vi "eyecat MAX v01.vi"() -> ()   [LabVIEW 2011]
doc: "This VI is an upgrade from the WIN 1_v4 that implements the ageing subrutine"
uses:
  Buttons/String output.ctl
  <vilib>/Utility/miscctls.llb/LVRowAndColumnTypeDef.ctl
  Buttons/Numeric control.ctl
  Buttons/String input.ctl
  Buttons/Numeric indicator.ctl
  Controls Win/Control 3.ctl
  <vilib>/Platform/TimedLoop/XDataNode/nitl_modes.ctl
  <vilib>/Platform/TimedLoop/XDataNode/timing_clust.ctl
  <vilib>/Platform/TimedLoop/XDataNode/wakeup.ctl
  <vilib>/Utility/file.llb/Write To Spreadsheet File (string).vi
  <vilib>/Utility/file.llb/Read From Spreadsheet File (string).vi
  <vilib>/Platform/TimedLoop/XDataNode/XDataNode.xnode
  <vilib>/regexp/Match Regular Expression.xnode
  <vilib>/Platform/TimedLoop/XDataNode/XDNodeRunTimeDep.lvlib
panel:
  out "Furnace temp 2":dbl
  out "output cluster":T2
  out "Full system?":bool
  out "Log interval (seconds)":T1
  in  "Flow rate Age":dbl
  in  "Inlet temp Age":dbl
  out "Stopped?":bool
  in  "Stop Cmd":T1
  out "Connected?":bool
  out "Error":dbl
  out "Iteration Duration":i64
  out "Finished Late? [i-1]":bool
  in  "stop TCP":bool
  in  "SO2 ppm":dbl
  out "Furnace temp 1":dbl
  out "stop 2":bool
  in  "Enum 1":i16=1
  in  "Acknowledge":bool
  out "Test number":u16
  out "Flag1":bool=TRUE
  out "EditPos Subc":T3
  out "Flag 2":bool=TRUE
  in  "Tab Control":T4(tab)
  out "Doors Unlocked":bool
  in  "Temperature Limit (°C)":T1=800.0 min=0.0 max=1200.0 step=1.0
  in  "Log Test Button":bool
  in  "File Name":T5
  in  "File Path":path=path "C:/DATA LOG"
  out "Fail":bool
  out "Pass":bool
  in  "Select Test Type":T6(radio)
  out "Standby":bool
  out "Doors Open":bool
  out "Extractor Fan On":bool
  out "Test In Progress":bool
  out "Cool Down":bool
  out "System Alarm":bool
  in  "Execute Leak Test Button":bool
  in  "Stop Test Button":bool
  in  "Start Test Button":bool
  in  "Advanced settings":bool
  in  "Inlet Temperature (°C)":T1=400.0 min=350.0 max=1000.0 step=1.0
  in  "Inlet LAMBDA Rich":T1=0.9 min=0.85 max=0.96 step=0.001
  in  "Inlet LAMBDA Lean":T1=1.2 min=1.02 max=3.0 step=0.001
  in  "Test Stop temperature (°C)":T1=300.0 min=100.0 max=1000.0 step=1.0
  in  "Test Start Temperature (°C)":T1=125.0 min=0.0 max=500.0 step=1.0
  in  "Furnace Ramp Rate (°C/min)":T1=15.0 min=1.0 max=50.0 step=0.1
  in  "NO:CO Ratio":T1=1.1 min=1.0 max=5.0 step=0.1
  in  "Inlet O2 (%)":T1=0.5 min=0.0 max=14.0 step=0.01
  in  "Inlet LAMBDA":T1=1.0 min=0.6 max=3.0 step=0.001
  out "Space Velocity (h-1)":T7
  out "Vol Flow @ STP (l/min)":T7
  in  "Test Flow Rate(g/s)":T1 min=0.0 max=100.0 step=0.01
  out "Sample Volume (litres)":T7
  in  "Number of Samples":T1=1.0 min=1.0 max=6.0 step=1.0
  in  "Sample Diameter (mm)":T1
  out "CO Theory (%)":T7 format="%#_3g"
  out "CO Theory (%)":T7 format="%#_3g"
  out "HC Theory (%)":T7
  in  "Sample Length (mm)":T1 min=0.0 step=0.5
  in  "NO ppm SW":dbl=500.0 caption="NO (ppm)" min=0.0 max=500.0 step=1.0
  in  "NO ppm Loff":T1 caption="NO ppm"
  in  "Delete sCycle":bool
  in  "Load sCycle":bool
  in  "Save sCycle":bool
  in  "Clear subcycle":bool
  in  "Clear Cycle Pattern":bool
  in  "Save Cycle":bool
  in  "Load Cycle":bool
  in  "Delete Cycle":bool
  out "Test Compiled":bool
  in  "Compile Test Button":bool
  in  "Sub-Cycle List":i32(listbox)=1
  in  "Cycle List":i32(listbox)=2
  out "Total Test Duration (hrs)":T8
  in  "Ageing Gas":enum32{"Radio Selection 1", "Radio Selection 2"}(radio)
  in  "Sub-Cycle Pattern":string[][](table) caption="Subcycle pattern"
  in  "Total Number of Cycles":T1=1.0 min=1.0 max=10000.0 step=1.0
  in  "Cycle Pattern":string[][](table)
  in  "Sub-Cycle Name":T5
  in  "Cycle Name":T5
  out "Heat Exchanger Temperatures (°C)":dynamicdata(graph)
  out "Flow Rate (g/s)":dynamicdata(graph)
  out "Sample Temperatures (°C)":dynamicdata(graph)
  out "System Temperatures (°C)":dynamicdata(graph)
  out "HC Concentration (ppm)":dynamicdata(graph)
  out "Lambda":dynamicdata(graph)
  out "M584L Upstream & Downstream":dynamicdata(graph)
  out "NO Concentration (ppm)":dynamicdata(graph)
  in  "Purge System":bool
  in  "Alarm ack":bool
  in  "Clear log":bool
  out "Table":string[][](table)
  out "Soft Alarm":bool
  out "Hard Alarm":bool
  # "Test Type"
  # "Test Commands"
  # "System Indicators"
  # "Leak Test"
  # "Catalyst Specification"
  # "Lightoff Settings"
  # "Furnace Lightoff Settings"
  # "Sweep Settings"
  # "CO/HC Lightoff Settings"
  # "0.96 < lambda < 0.85"
  # "1.02< lambda < 1.6"
  # "350 < Tinlet < 1000"
  # "NO Lightoff Settings"
  # "Flow Specification"
  # "Cycle Compiled"
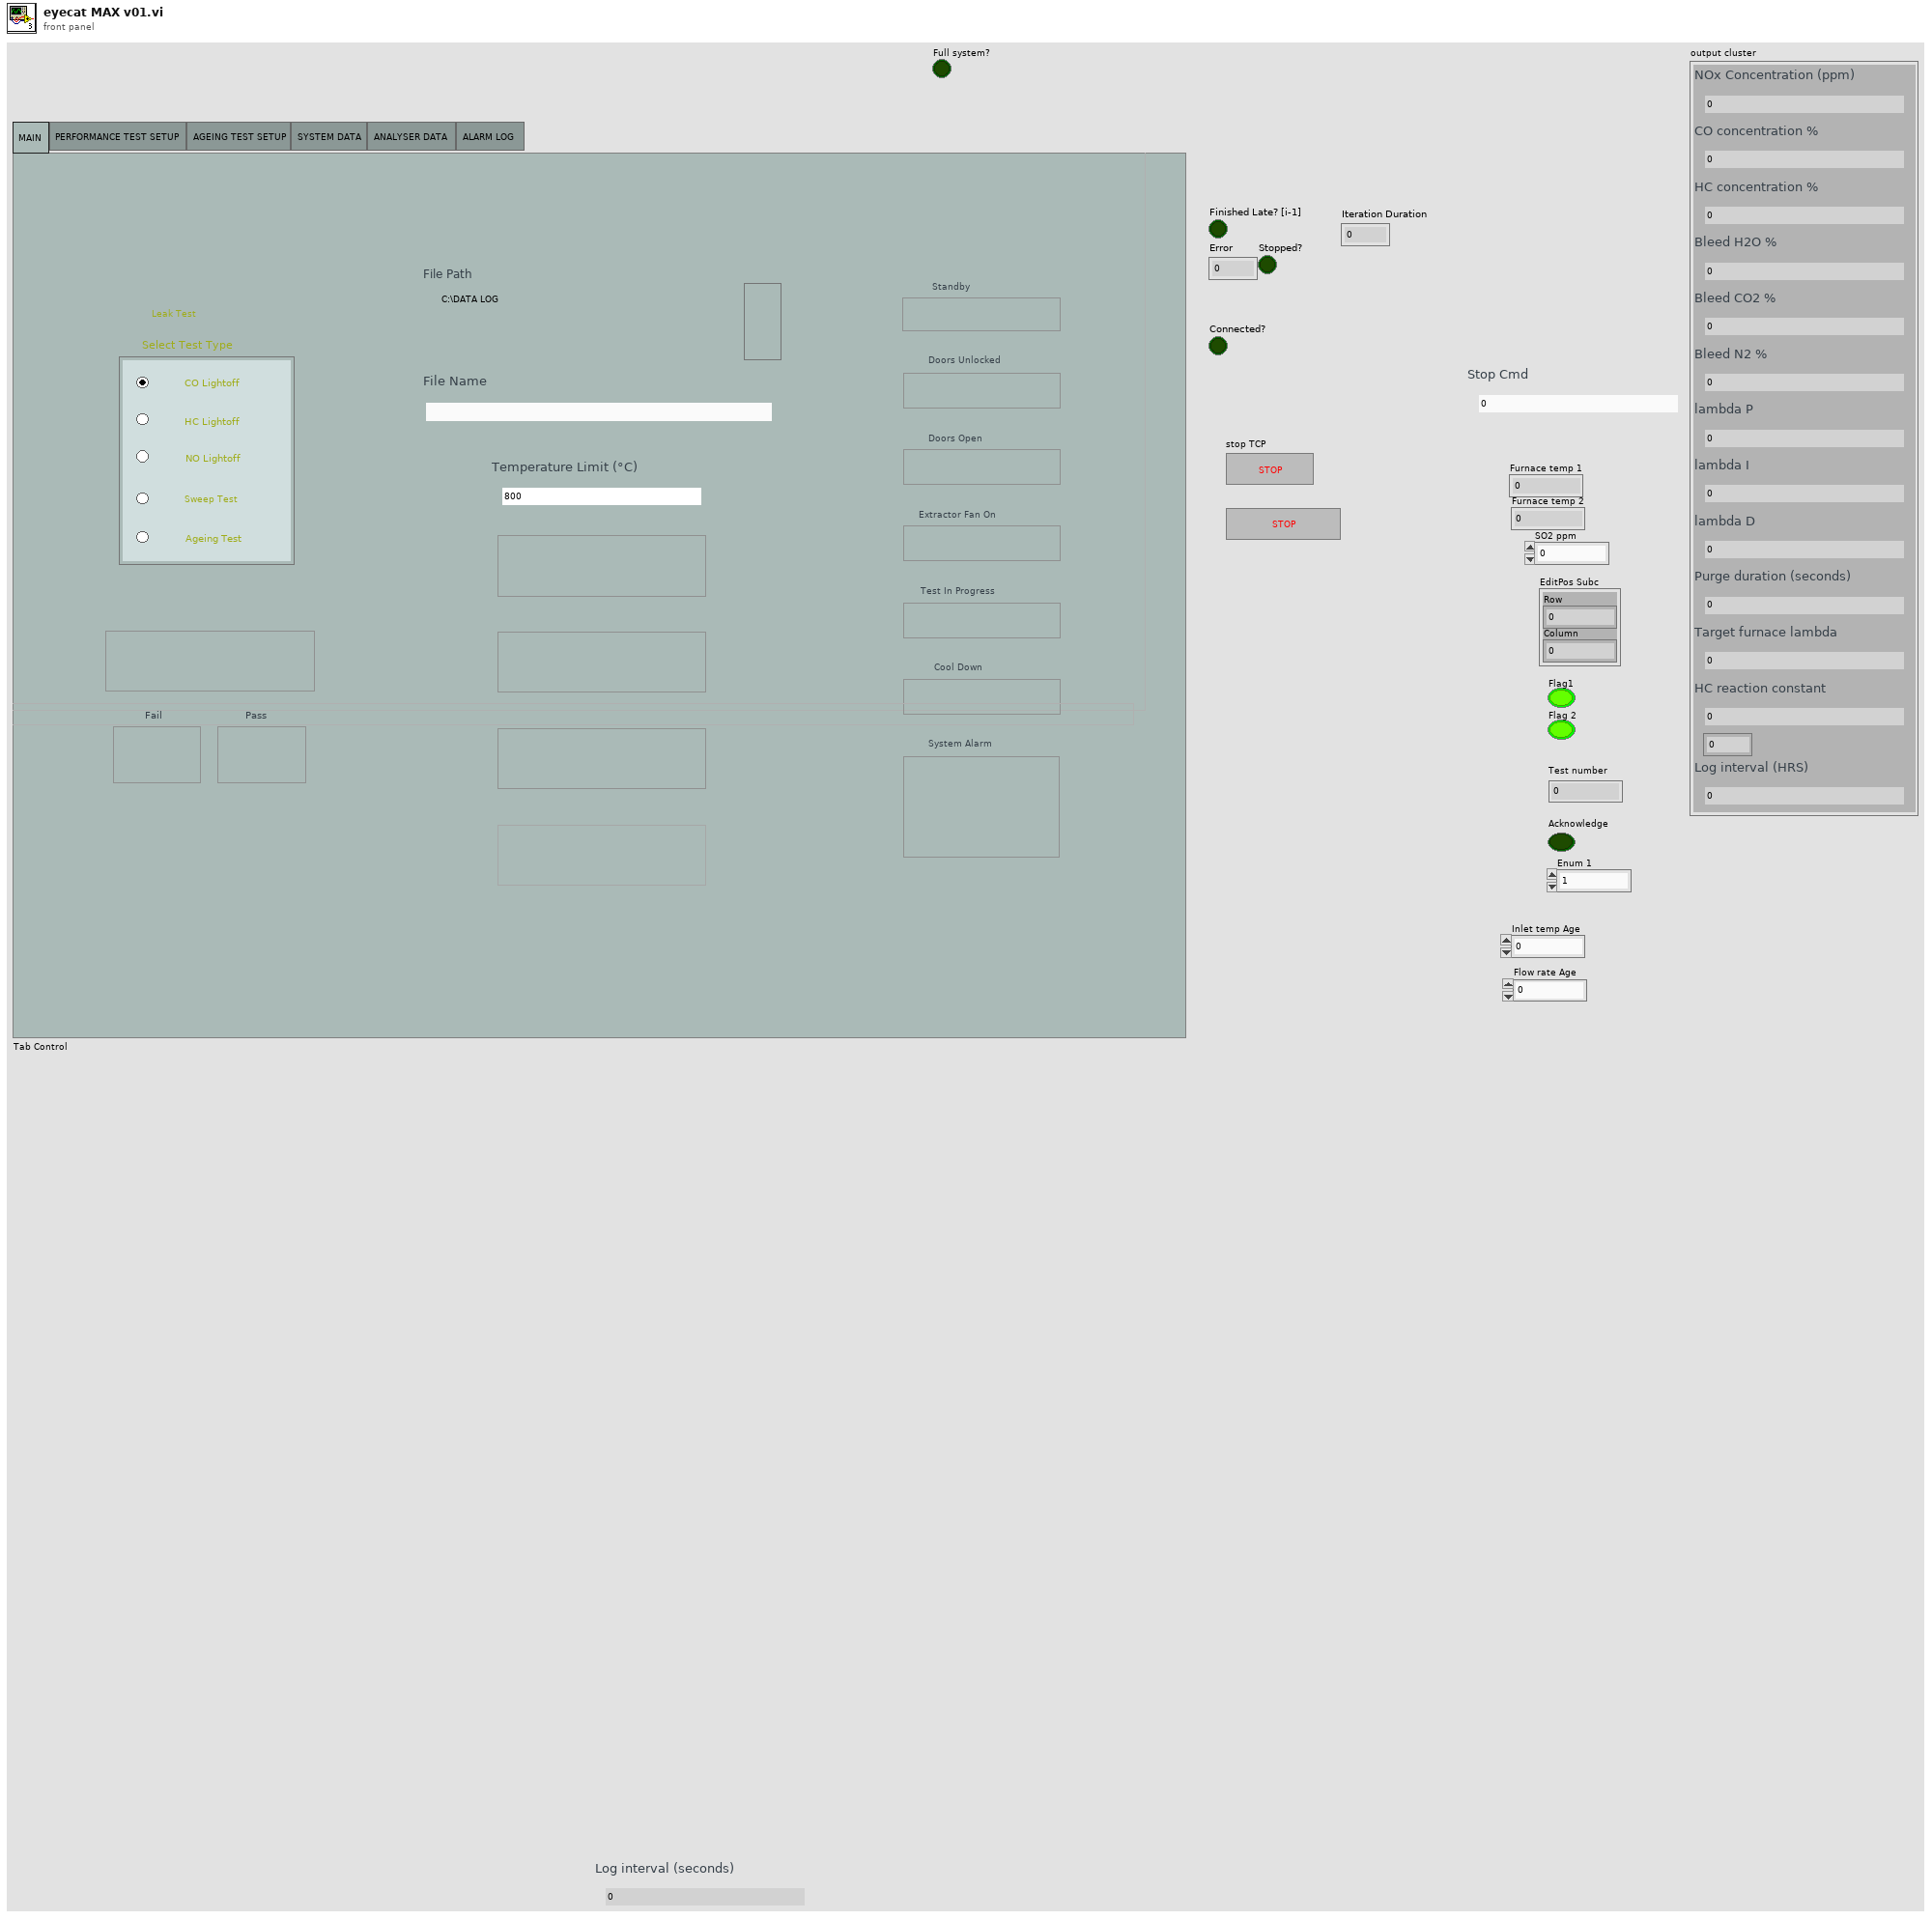
[diagram p1: front panel]
types:
  T1 = typedef "Numeric control.ctl" = dbl
  T2 = cluster{"NOx Concentration (ppm)":T1, "CO concentration %":T1, "HC concentration %":T1, "Bleed H2O %":T1, "Bleed CO2 %":T1, "Bleed N2 %":T1, "lambda P":T1, "lambda I":T1, "lambda D":T1, "Purge duration (seconds)":T1, "Target furnace lambda":T1, "HC reaction constant":T1, i16, "Log interval (HRS)":T1}
  T3 = typedef "LVRowAndColumnTypeDef.ctl" = cluster{"Row":i32, "Column":i32}
  T4 = enum32{"MAIN", "PERFORMANCE TEST SETUP", "AGEING TEST SETUP", "SYSTEM DATA", "ANALYSER DATA", "ALARM LOG"}
  T5 = typedef "String input.ctl" = string
  T6 = enum32{"CO Lightoff", "HC Lightoff", "NO Lightoff", "Sweep Test", "Ageing Test"}
  T7 = typedef "Numeric indicator.ctl" = dbl
  T8 = typedef "String output.ctl" = string
  T9 = typedef "XDNodeRunTimeDep.lvlib/nitl_modes.ctl" = enum32{"No Change", "Process missed periods, maintain original phase", "Discard missed periods, maintain original phase", "Process missed periods, ignore original phase", "Discard missed periods, ignore original phase"}
  T10 = typedef "Control 3.ctl" = enum16{"main", "start test", "save subc", "load subc", "delete subc", "clear table 1", "update list 1", "save cycle", "load cycle", "delete cycle", "clear table 2", "update list 2", "calc HC CO", "Total time calc", "update Cycle pattern ", "load cycle name", "convert to num", "load test array", "check scycle name", "check cycle name", "Multigas connect", "Multigas disconnect"}
  T11 = typedef "XDNodeRunTimeDep.lvlib/timing_clust.ctl" = cluster{"Expected End [f-1]":u64, "Actual End [f-1]":u64, "Finished Late? [f-1]":bool, "Expected End [i-1]":u64, "Actual End [i-1]":u64, "Finished Late? [i-1]":bool, "Expected Start [i]":u64, "Actual Start [i]":u64, "Expected Start [f]":u64, "Actual Start [f]":u64, "Source Name":string, "Structure Name":string, "Period":i64, "Deadline":i64, "Offset":i64, "Start":i64, "Priority":i32, "Timeout":i32, "Mode":T9, "Wakeup Reason":T12, "Error":errorcluster, "Source Type":string, "Secondary Source Type":string, "Global End Time":u64, "Global Start Time":u64, "Frame Duration":u64, "Iteration Duration":u64, "Assigned CPU":i32, "I/O Scan Engine Mode":u32}
  T12 = typedef "XDNodeRunTimeDep.lvlib/wakeup.ctl" = enum32{"Normal", "Aborted", "Asynchronous wakeup", "Timing source error", "Timed loop error", "Timeout"}
  T13 = enum8{"Enabled", "Disabled", "Disabled and Grayed Out"}
  T14 = cluster{"NOx Concentration (ppm)":T1, "CO concentration %":T1, "HC concentration %":T1, "Bleed H2O %":T1, "Bleed CO2 %":T1, "Bleed N2 %":T1, "lambda P":T1, "lambda I":T1, "lambda D":T1, "Purge duration (seconds)":T1, "Target furnace lambda":T1, "HC reaction constant":T1, "Full System?":i16, "Log interval (HRS)":T1}
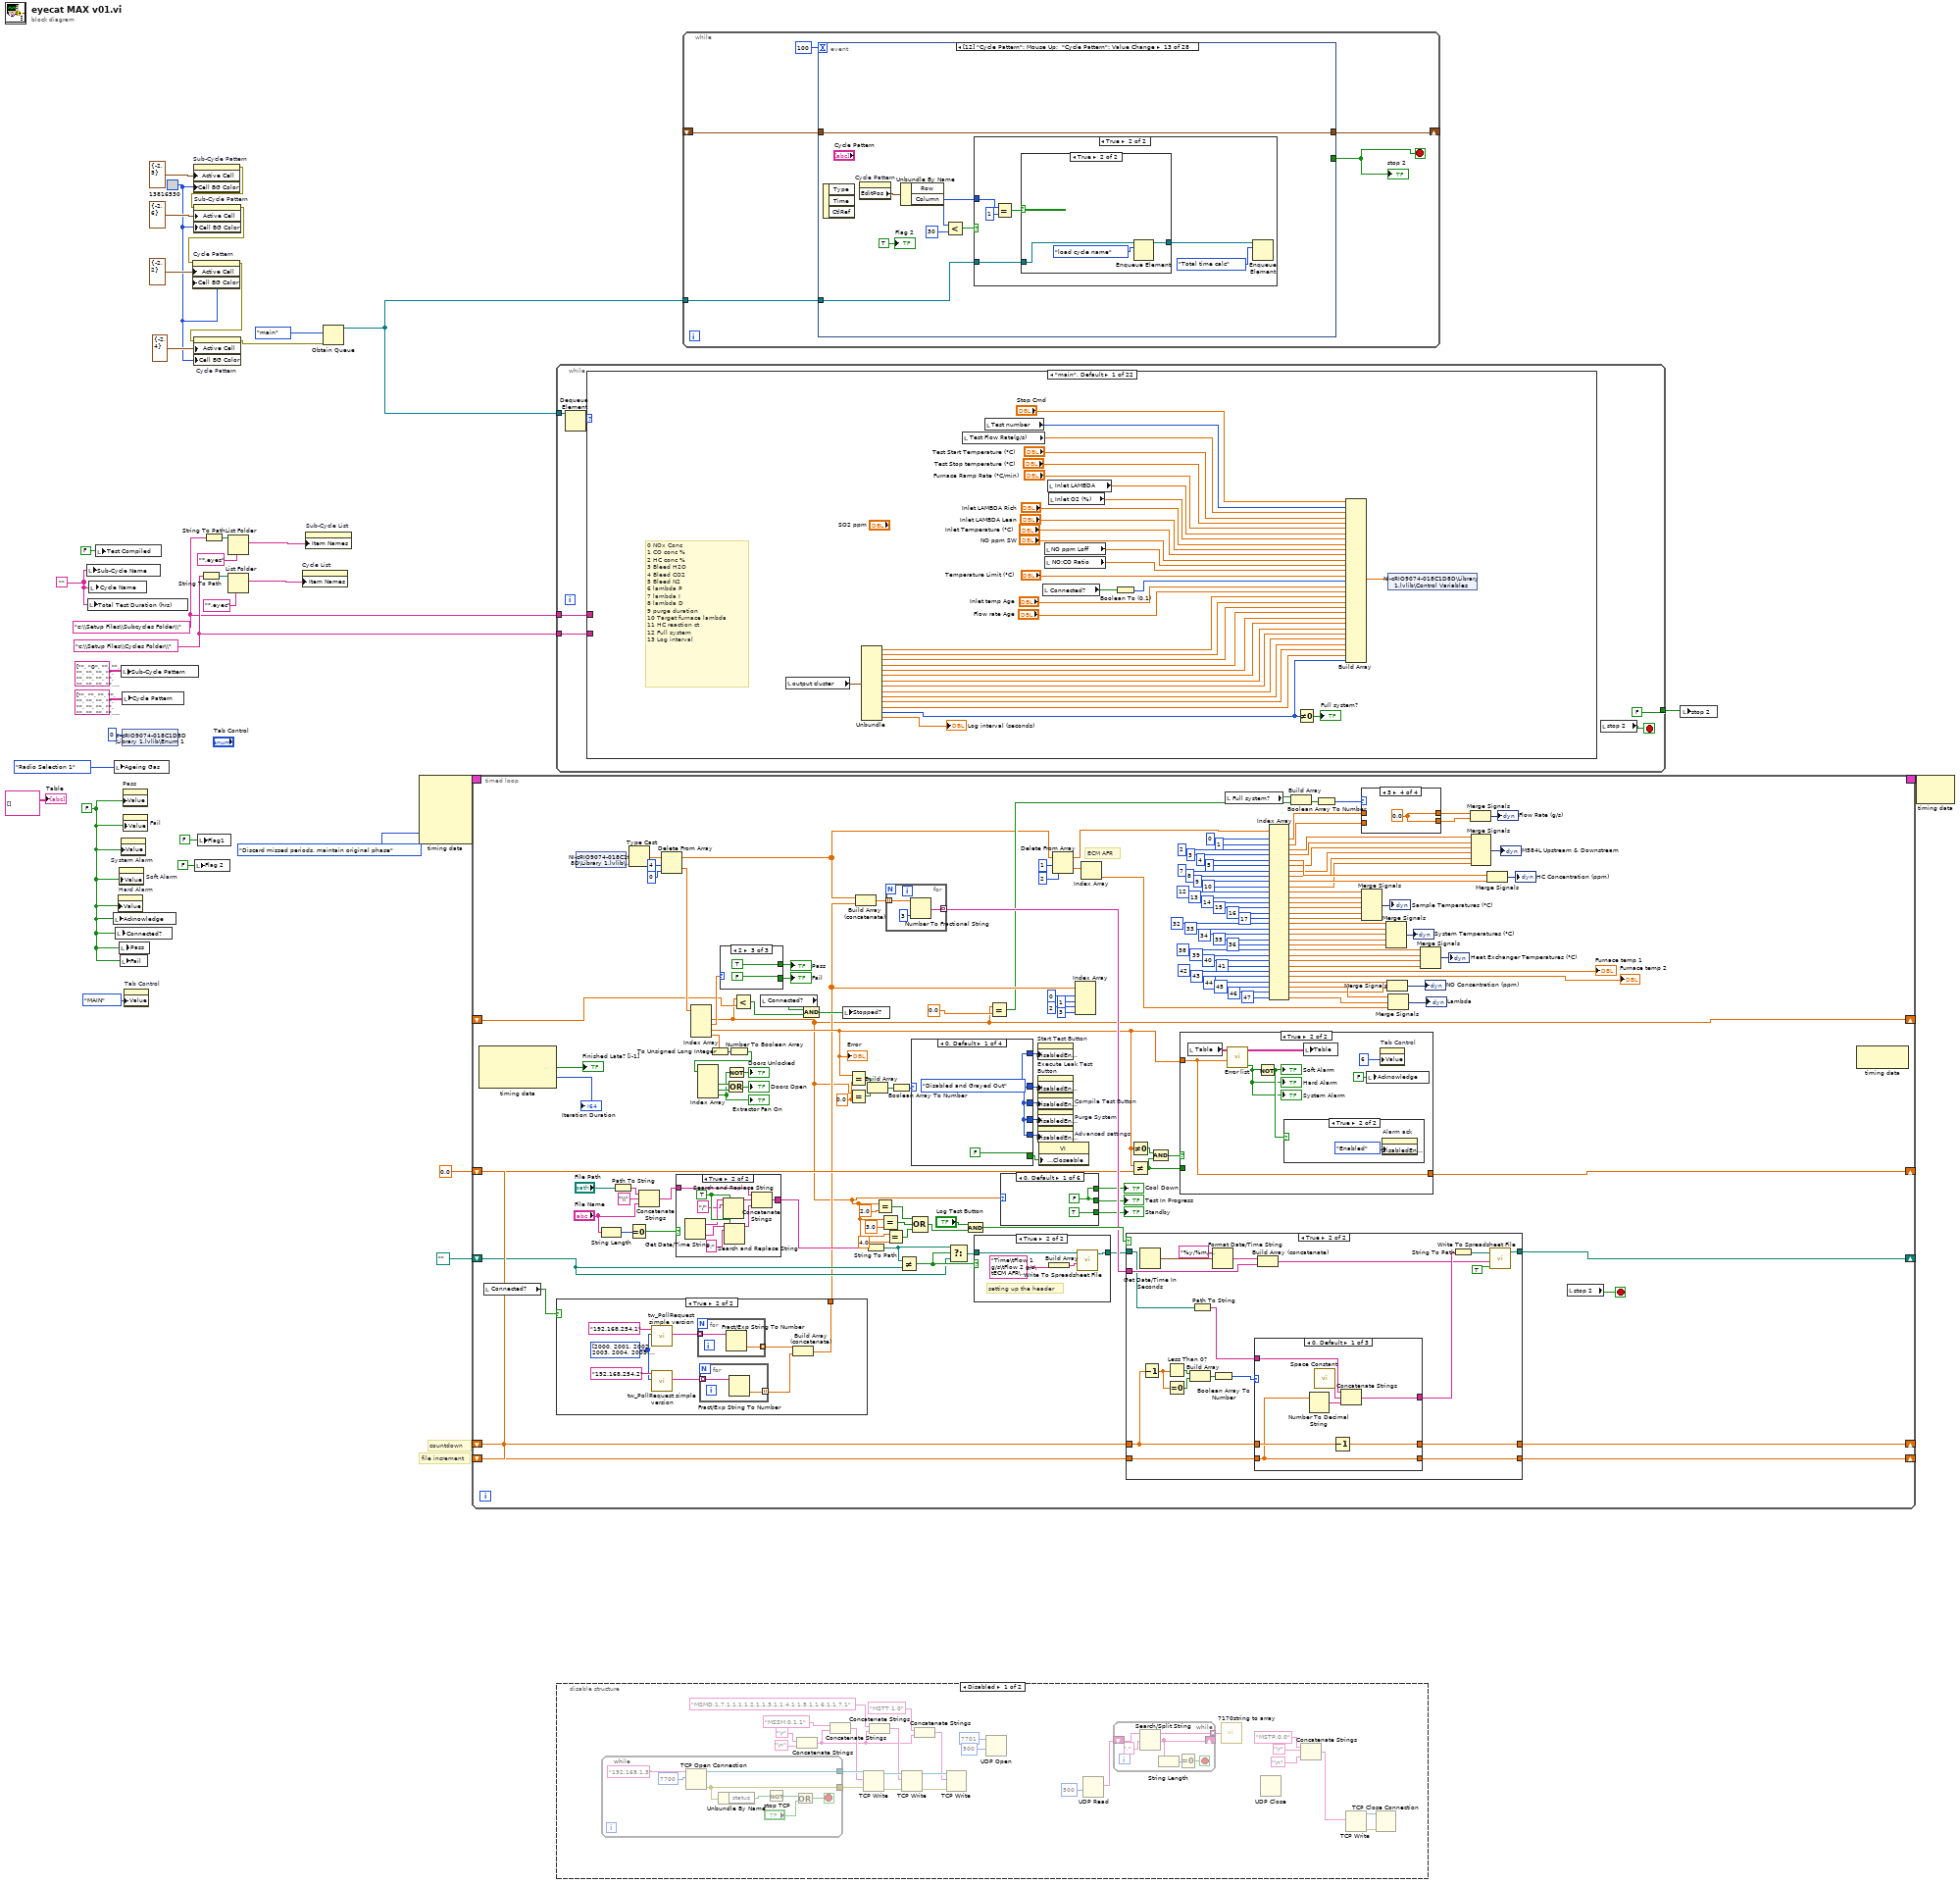
[diagram p0: block diagram]
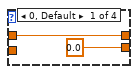
[diagram p3: hidden frame]
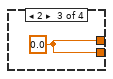
[diagram p5: hidden frame]
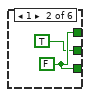
[diagram p7: hidden frame]
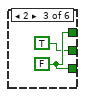
[diagram p8: hidden frame]
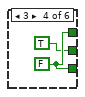
[diagram p9: hidden frame]
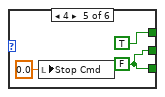
[diagram p10: hidden frame]
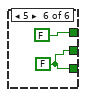
[diagram p11: hidden frame]
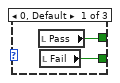
[diagram p12: hidden frame]
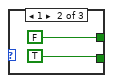
[diagram p13: hidden frame]
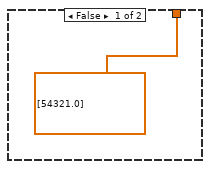
[diagram p14: hidden frame]
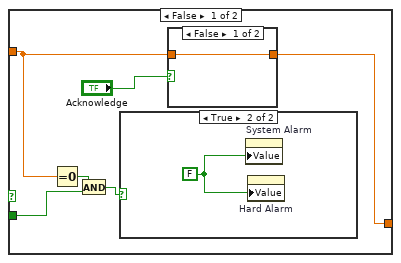
[diagram p15: hidden frame]
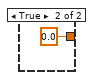
[diagram p16: hidden frame]
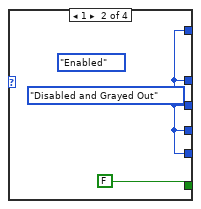
[diagram p19: hidden frame]
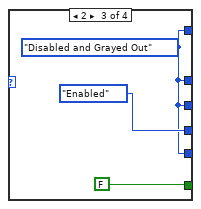
[diagram p20: hidden frame]
diagram:
  w2 = FALSE
  w1 = 0.0 ("y")
  w18 = ""
  w21 = "c:\\Setup Files\\Cycles Folder\\"
  w27 = u32 13816530
  w19 = "c:\\Setup Files\\Subcycles Folder\\"
  # "file increment"
  # "countdown"
  n1 = local write "Sub-Cycle Name"(w18) -> ()
  n2 = local write "Total Test Duration (hrs)"(w18) -> ()
  n3 = local write "Cycle Name"(w18) -> ()
  n4 = local write "Test Compiled"(FALSE ("Cycle Compiled")) -> ()
  n5 = local write "Acknowledge"(w2) -> ()
  n6 = local write "Ageing Gas"(enum32{"Radio Selection 1", "Radio Selection 2"}."Radio Selection 1" ("Ageing Gas")) -> ()
  n7 = local write "Connected?"(w2) -> ()
  n8 = property on="Hard Alarm" class="Bool (strict)"("Value"=w2) -> ()  [unwired: 2 in, 2 out]
  n9 = property on="Soft Alarm" class="Bool (strict)"("Value"=w2) -> ()  [unwired: 2 in, 2 out]
  n10 = local write "Pass"(w2) -> ()
  n11 = local write "Fail"(w2) -> ()
  n12 = local write "Sub-Cycle Pattern"(string[][] [["", "0", "", "", "", "", "", "", "", "", "", "", ""], ["", "", "", "", "", "", "", "", "", "", "", "", ""], ["", "", "", "", "", "", "", "", "", "", "", "", ""], ["", "", "", "", "", "", "", "", "", "", "", "", ""], ["", "", "", "", "", "", "", "", "", "", "", "", ""], ["", "", "", "", "", "", "", "", "", "", "", "", ""], ["", "", "", "", "", "", "", "", "", "", "", "", ""], ["", "", "", "", "", "", "", "", "", "", "", "", ""], ["", "", "", "", "", "", "", "", "", "", "", "", ""], ["", "", "", "", "", "", "", "", "", "", "", "", ""], ["", "", "", "", "", "", "", "", "", "", "", "", ""], ["", "", "", "", "", "", "", "", "", "", "", "", ""], ["", "", "", "", "", "", "", "", "", "", "", "", ""], ["", "", "", "", "", "", "", "", "", "", "", "", ""], ["", "", "", "", "", "", "", "", "", "", "", "", ""], ["", "", "", "", "", "", "", "", "", "", "", "", ""], ["", "", "", "", "", "", "", "", "", "", "", "", ""], ["", "", "", "", "", "", "", "", "", "", "", "", ""], ["", "", "", "", "", "", "", "", "", "", "", "", ""], ["", "", "", "", "", "", "", "", "", "", "", "", ""], ["", "", "", "", "", "", "", "", "", "", "", "", ""], ["", "", "", "", "", "", "", "", "", "", "", "", ""], ["", "", "", "", "", "", "", "", "", "", "", "", ""], ["", "", "", "", "", "", "", "", "", "", "", "", ""], ["", "", "", "", "", "", "", "", "", "", "", "", ""], ["", "", "", "", "", "", "", "", "", "", "", "", ""], ["", "", "", "", "", "", "", "", "", "", "", "", ""], ["", "", "", "", "", "", "", "", "", "", "", "", ""], ["", "", "", "", "", "", "", "", "", "", "", "", ""], ["", "", "", "", "", "", "", "", "", "", "", "", ""], ["", "", "", "", "", "", "", "", "", "", "", "", ""]]) -> ()
  n13 = property on="System Alarm" class="Bool (strict)"("Value"=w2) -> ()  [unwired: 2 in, 2 out]
  n14 = local write "Cycle Pattern"(string[][] [["", "", "", "", ""], ["", "", "", "", ""], ["", "", "", "", ""], ["", "", "", "", ""], ["", "", "", "", ""], ["", "", "", "", ""], ["", "", "", "", ""], ["", "", "", "", ""], ["", "", "", "", ""], ["", "", "", "", ""], ["", "", "", "", ""], ["", "", "", "", ""], ["", "", "", "", ""], ["", "", "", "", ""], ["", "", "", "", ""], ["", "", "", "", ""], ["", "", "", "", ""], ["", "", "", "", ""], ["", "", "", "", ""], ["", "", "", "", ""], ["", "", "", "", ""], ["", "", "", "", ""], ["", "", "", "", ""], ["", "", "", "", ""], ["", "", "", "", ""], ["", "", "", "", ""], ["", "", "", "", ""], ["", "", "", "", ""], ["", "", "", "", ""], ["", "", "", "", ""], ["", "", "", "", ""]]) -> ()
  n15 = shared-variable "NI-cRIO9074-018C1D8D\\Library 1.lvlib\\Enum 1"(u16 0 ("Enum 1")) -> ()  [unwired: 1 in, 1 out]
  n16 = property on="Pass" class="Bool (strict)"("Value"=w2) -> ()  [unwired: 2 in, 2 out]
  n17 = property on="Fail" class="Bool (strict)"("Value"=w2) -> ()  [unwired: 2 in, 2 out]
  n18 = property on="Tab Control" class="TabCtl (strict)"("Value"=T4."MAIN" ("Tab Control")) -> ()  [unwired: 2 in, 2 out]
  n19 = property on="Sub-Cycle Pattern" class="Tbl (strict)"("Active Cell"=T3 {"Row"=-2, "Column"=5} ("Active Cell:Active Cell"), "Cell BG Color"=w27) -> (error out=w32:errorcluster)  [unwired: 2 in, 1 out]
  n20 = property on="Sub-Cycle Pattern" class="Tbl (strict)"(error in=w32, "Active Cell"=T3 {"Row"=-2, "Column"=6} ("Active Cell:Active Cell"), "Cell BG Color"=w27) -> (error out=w31:errorcluster)  [unwired: 1 in, 1 out]
  n21 = property on="Cycle Pattern" class="Tbl (strict)"(error in=w31, "Active Cell"=T3 {"Row"=-2, "Column"=2} ("Active Cell:Active Cell"), "Cell BG Color"=w27) -> (error out=w29:errorcluster)  [unwired: 1 in, 1 out]
  n22 = property on="Cycle Pattern" class="Tbl (strict)"(error in=w29, "Active Cell"=T3 {"Row"=-2, "Column"=4} ("Active Cell:Active Cell"), "Cell BG Color"=w27) -> (error out=w26:errorcluster)  [unwired: 1 in, 1 out]
  n23 = local write "Flag 2"(FALSE) -> ()
  n24 = local write "Flag1"(FALSE) -> ()
  n25 = String To Path(string=w21) -> (path=w22:path)
  n26 = String To Path(string=w19) -> (path=w24:path)
  n27 = List Folder(path=w22, pattern="*.eyec") -> (filenames=w23:string[])  [unwired: 2 in, 3 out]
  n28 = List Folder(path=w24, pattern="*.eyes") -> (filenames=w25:string[])  [unwired: 2 in, 3 out]
  n29 = property on="Cycle List" class="LstBox (strict)"("Item Names"=w23) -> ()  [unwired: 2 in, 2 out]
  n30 = property on="Sub-Cycle List" class="LstBox (strict)"("Item Names"=w25) -> ()  [unwired: 2 in, 2 out]
  n31 = Obtain Queue(element data type=Control_3."main" ("Enum"), error in (no error)=w26) -> (queue out=w35:refnum<queue>)  [unwired: 3 in, 2 out]
  n32 = node-c288(nitl_modes."Discard missed periods, maintain original phase" ("Mode")) -> (w7:T11)  [unwired: 4 in]
  n33 = timed-loop {
    timing: w7 -> [_]
    timing-out: [_] -> w6
    shift-right: [w168] -> _
    shift-left: path "" -> [w170]
    shift-right: [w119] -> _
    shift-left: w1 -> [w169]
    shift-right: [w38] -> _
    shift-left: _ -> [w133]
    shift-right: [w108] -> _
    shift-left: w1 -> [w112]
    shift-right: [w109] -> _
    shift-left: w1 -> [w111]
    stop <- w167 stop-if-true
    w150 = 0.0 ("y")
    # "ECM AFR"
    n34 = node-c288() -> (→"Finished Late? [i-1]":bool, →"Iteration Duration":i64)  [unwired: 1 in, 1 out]
    n35 = local read "Connected?"() -> (w156:bool)
    n36 = case shown="True" w156 {
      tunnel: [dbl[] [54321.0] ("Output") w235] -> w107
      frame False {
      }
      frame True {
        w238 = i32[] [2000, 2001, 2002, 2003, 2004, 2005, 2006, 2007, 2008, 2009, 2010, 2011, 2012, 2013, 2014] ("EVID list")
        n37 = call <userlib>:"tw_PollRequest simple version.vi"("EVID list"=w238, "IP_ADD [127.0.0.1]"="192.168.254.1") -> ("values out"=w241:string[])  [unwired: 7 in, 2 out]
        n38 = call <userlib>:"tw_PollRequest simple version.vi"("EVID list"=w238, "IP_ADD [127.0.0.1]"="192.168.254.2") -> ("values out"=w240:string[])  [unwired: 7 in, 2 out]
        n39 = for {
          tunnel: [w246] -> w236 mode=indexing
          tunnel: w241 -> [w245] mode=indexing
          n40 = Fract/Exp String To Number(string=w245) -> (number=w246:dbl)  [unwired: 3 in, 1 out]
        }
        n41 = for {
          tunnel: [w244] -> w237 mode=indexing
          tunnel: w240 -> [w243] mode=indexing
          n42 = Fract/Exp String To Number(string=w243) -> (number=w244:dbl)  [unwired: 3 in, 1 out]
        }
        n43 = Build Array (concatenate)(w236, w237) -> (w235:dbl[])
      }
    }
    n44 = shared-variable "NI-cRIO9074-018C1D8D\\Library 1.lvlib\\DATA"() -> (w166:dbl[])  [unwired: 1 in, 1 out]
    n45 = String Length(string="File Name") -> (length=w124:i32)
    n46 = Path To String(path="File Path") -> (string=w126:string)
    n47 = Equal To 0?(x=w124) -> (x = 0?=w122:bool)
    n48 = Type Cast(type=w166, x=w166) -> (*(type *) &x=w179:dbl[])
    n49 = Concatenate Strings(w126, "\\" ("string"), "File Name") -> (w121:string)
    n50 = Delete From Array(array=w179, length=4, index=0) -> (deleted portion=w176:dbl[], array with subset deleted=w48:dbl[])
    n51 = case shown="True" w122 {
      tunnel: [w205 w213] -> w110
      tunnel: w121 -> [w205 w214]
      frame False {
      }
      frame True {
        w211 = TRUE ("replace all? (F)")
        n52 = Get Date/Time String() -> (date string=w209:string, time string=w210:string)  [unwired: 3 in]
        n53 = Search and Replace String(replace all?=w211, input string=w209, search string="/") -> (result string=w212:string)  [unwired: 5 in, 3 out]
        n54 = Search and Replace String(replace all?=w211, input string=w210, search string=":") -> (result string=w206:string)  [unwired: 5 in, 3 out]
        n55 = Concatenate Strings(w214, w212, w206) -> (w213:string)
      }
    }
    n56 = Index Array(array=w176) -> (element #1=w38:dbl, element #2=w139:dbl, element #3=w140:dbl, element #4=w132:dbl)  [unwired: 4 in]
    "Error" <- w140
    n57 = To Unsigned Long Integer(number=w132) -> (unsigned 32bit integer=w131:u32)
    n58 = case shown="2" w139 {
      tunnel: [w228 TRUE FALSE] -> w138
      tunnel: [w229 FALSE TRUE] -> w137
      frame 0, Default {
        n59 = local read "Pass"() -> (w229:bool)
        n60 = local read "Fail"() -> (w228:bool)
      }
      frame 1 {
      }
      frame 2 {
      }
    }
    "Pass" <- w137
    "Fail" <- w138
    n61 = Number To Boolean Array(number=w131) -> (Boolean array=w155:bool[])
    n62 = Index Array(array=w155) -> (element #2=w153:bool, element #3=w152:bool, element #4=w128:bool)  [unwired: 4 in, 1 out]
    "Extractor Fan On" <- w128
    n63 = Or(x=w153, y=w152) -> (x .or. y?=→"Doors Open":bool)
    n64 = Not(x=w128) -> (.not. x?=→"Doors Unlocked":bool)
    n65 = Less?(x=w38, y=w133) -> (x < y?=w130:bool)
    n66 = local read "Connected?"() -> (w129:bool)
    n67 = And(x=w129, y=w130) -> (x .and. y?=w118:bool)
    n68 = local write "Stopped?"(w118) -> ()
    n69 = Equal?(x=w140, y=w150) -> (x = y?=w148:bool)
    n70 = Equal?(x=w38, y=w150) -> (x = y?=w147:bool)
    n71 = Build Array (concatenate)(w48, w107) -> (w172:dbl[])
    n72 = String To Path(string=w110) -> (path=w120:path)
    n73 = Build Array(w148, w147) -> (w146:bool[])
    n74 = Equal?(x=w38, y=2.0) -> (x = y?=w50:bool)
    n75 = Equal?(x=w38, y=3.0) -> (x = y?=w41:bool)
    n76 = Equal?(x=w38, y=4.0) -> (x = y?=w39:bool)
    n77 = for {
      tunnel: w172 -> [w279] mode=indexing
      tunnel: [w278] -> w183 mode=indexing
      n78 = Number To Fractional String(number=w279, precision (6)=i16 3) -> (F-format string=w278:string)  [unwired: 2 in]
    }
    n79 = Boolean Array To Number(Boolean array=w146) -> (number=w145:u32)
    n80 = Not Equal?(x=w120, y=w170) -> (x != y?=w181:bool)
    n81 = case shown="0, Default" w145 {
      tunnel: [w265 w267 w269 w272] -> w149
      tunnel: [w265 w267 w269 w272] -> w144
      tunnel: [w265 w267 w269 w272] -> w143
      tunnel: [w265 w267 T13."Enabled" ("Disabled") w272] -> w142
      tunnel: [w265 w267 w269 w272] -> w141
      tunnel: [FALSE FALSE FALSE TRUE] -> w117
      frame 0, Default {
        w265 = T13."Disabled and Grayed Out" ("Disabled")
      }
      frame 1 {
        (unwired) T13."Enabled" ("Disabled")
        w267 = T13."Disabled and Grayed Out" ("Disabled")
      }
      frame 2 {
        w269 = T13."Disabled and Grayed Out" ("Disabled")
      }
      frame 3 {
        w272 = T13."Enabled" ("Disabled")
        (unwired) T13."Disabled and Grayed Out" ("Disabled")
      }
    }
    n82 = Compound Arithmetic op=OR(w50, w41, w39) -> (w49:bool)
    n83 = Select(t=w120, s=w181, f=w170) -> (s? t:f=w182:path)
    n84 = And(x="Log Test Button", y=w49) -> (x .and. y?=w198:bool)
    n85 = case shown="True" w181 {
      tunnel: w182 -> [w273 w277]
      tunnel: [w273 w276] -> w180
      frame False {
      }
      frame True {
        # "setting up the header"
        n86 = Build Array("Time\tFlow 1 g/s\tFlow 2 g/s\tECM AFR\tCO2 U %\tCO U %\tHC U ppm\tO2 U %\tNO U ppm\tCO2 D %\tCO D %\tHC D ppm\tO2 D %\tNO D ppm\tTC1X\tTC2A\tTCY\tTC4B\tTC5\tTC6\tTC7\tTC8\tTC9\tTC10\tTC11\tTC12\tTC13\tTC14\tTC15\tTC16\tTC17\tTC18\tTC19\tTC20\tTC Vent 1\tTC Vent 2\tTC Fan B1\tTC Fan B2\tTC Cab\tTC Ex A\tTC Ex B\tTC Ex C\tTC Ex D\tTC Furn 1\tTC Furn 2\tNOX 1 ppm\tNLambda 1\tNOX 2 ppm\tNLambda 2\tEGO 1\tEGO 2\tEGO 3\tEGO 4\tCO2 U %\tCO U %\tHC U ppm\tO2 U %\tNO U ppm\tCO2 D %\tCO D %\tHC D ppm\tO2 D %\tNO D ppm\r\n" ("Heading string 2")) -> (w275:string[])
        n87 = call-poly <vilib>:"Write To Spreadsheet File.vi"("1D data"=w275, "file path (dialog if empty)"=w277) -> ("new file path (Not A Path if cancelled)"=w276:path)  [unwired: 6 in]
      }
    }
    n88 = Equal?(x=w38, y=0.0) -> (x = y?=w104:bool)
    n89 = case shown="0, Default" w38 {
      tunnel: [w215 w218 w220 w222 TRUE FALSE] -> w136
      tunnel: [w215 TRUE TRUE TRUE w224 w226] -> w135
      tunnel: [TRUE w218 w220 w222 w224 w226] -> w134
      frame 0, Default {
        w215 = FALSE
      }
      frame 1 {
        w218 = FALSE
      }
      frame 2 {
        w220 = FALSE
      }
      frame 3 {
        w222 = FALSE
      }
      frame 4 {
        w224 = FALSE
        n90 = local write "Stop Cmd"(T1 0.0 ("Stop Cmd")) -> ()
      }
      frame 5 {
        w226 = FALSE
      }
    }
    "Cool Down" <- w136
    "Test In Progress" <- w135
    "Standby" <- w134
    n91 = property on="Start Test Button" class="Bool"("DisabledEnum"=w149) -> ()  [unwired: 2 in, 2 out]
    n92 = property on="Execute Leak Test Button" class="Bool"("DisabledEnum"=w144) -> ()  [unwired: 2 in, 2 out]
    n93 = property on="Compile Test Button" class="Bool"("DisabledEnum"=w143) -> ()  [unwired: 2 in, 2 out]
    n94 = property on="Purge System" class="Bool"("DisabledEnum"=w142) -> ()  [unwired: 2 in, 2 out]
    n95 = property on="Advanced settings" class="Bool"("DisabledEnum"=w141) -> ()  [unwired: 2 in, 2 out]
    n96 = property class="VI"("Front Panel.Closeable"=w117) -> ()  [unwired: 2 in, 2 out]
    n97 = Delete From Array(array=w48, length=1, index=2) -> (deleted portion=w45:dbl[], array with subset deleted=w43:dbl[])
    n98 = Index Array(array=w107, index #1=0 ("index"), index #2=1 ("index"), index #3=2 ("index"), index #4=3 ("index")) -> ()  [unwired: 4 out]
    n99 = Index Array(array=w45) -> (element=w44:dbl)  [unwired: 1 in]
    n100 = case shown="True" w198 {
      tunnel: w180 -> [w283 w291]
      tunnel: [w283 w303] -> w168
      tunnel: w183 -> [_ w299]
      tunnel: w112 -> [_ w292]
      tunnel: w111 -> [w282 w287]
      tunnel: [w282 w289] -> w109
      tunnel: [w281 w288] -> w108
      frame False {
        n101 = local read "Log interval (seconds)"() -> (w281:T1)
      }
      frame True {
        n102 = Get Date/Time In Seconds() -> (seconds since 1Jan1904=w300:timestamp)
        n103 = Decrement(x=w292) -> (x-1=w293:T1)
        n104 = Less Than 0?(x=w293) -> (x < 0?=w294:bool)
        n105 = Equal To 0?(x=w293) -> (x = 0?=w295:bool)
        n106 = Build Array(w294, w295) -> (w296:bool[])
        n107 = Path To String(path=w291) -> (string=w286:string)
        n108 = Format Date/Time String(time format string (%c)="%y/%m/%d %H:%M:%S", seconds (now)=w300) -> (date/time string=w301:string)  [unwired: 1 in]
        n109 = Boolean Array To Number(Boolean array=w296) -> (number=w297:u32)
        n110 = case shown="0, Default" w297 {
          tunnel: w292 -> [w310 w311 _]
          tunnel: [w309 w311 w314] -> w288
          tunnel: w286 -> [w308 w313 w317]
          tunnel: [w305 w313 w315] -> w290
          tunnel: [w304 w312 w316] -> w289
          tunnel: w287 -> [w304 w312 w320]
          frame 0, Default {
            n111 = Number To Decimal String(number=w304) -> (decimal integer string=w306:string)  [unwired: 1 in]
            n112 = call <vilib>:"Space Constant.vi"() -> ("String"=w307:string)
            n113 = Decrement(x=w310) -> (x-1=w309:T1)
            n114 = Concatenate Strings(w308, w307, w306) -> (w305:string)
          }
          frame 1 {
          }
          frame 2 {
            n115 = local read "Log interval (seconds)"() -> (w314:T1)
            n116 = Increment(x=w320) -> (x+1=w316:dbl)
            n117 = Number To Decimal String(number=w316) -> (decimal integer string=w318:string)  [unwired: 1 in]
            n118 = call <vilib>:"Space Constant.vi"() -> ("String"=w319:string)
            n119 = Concatenate Strings(w317, w319, w318) -> (w315:string)
          }
        }
        n120 = Build Array (concatenate)(w301, w299) -> (w285:string[])
        n121 = String To Path(string=w290) -> (path=w284:path)
        n122 = call-poly <vilib>:"Write To Spreadsheet File.vi"("append to file? (new file:F)"=TRUE, "1D data"=w285, "file path (dialog if empty)"=w284) -> ("new file path (Not A Path if cancelled)"=w303:path)  [unwired: 5 in]
      }
    }
    n123 = Not Equal To 0?(x=w140) -> (x != 0?=w174:bool)
    n124 = Not Equal?(x=w140, y=w169) -> (x != y?=w173:bool)
    n125 = And(x=w174, y=w173) -> (x .and. y?=w175:bool)
    n126 = case shown="True" w175 {
      tunnel: w140 -> [w248 w259]
      tunnel: w173 -> [w251 _]
      tunnel: [w247 w259] -> w119
      frame False {
        n127 = Equal To 0?(x=w248) -> (x = 0?=w252:bool)
        n128 = And(x=w252, y=w251) -> (x .and. y?=w250:bool)
        n129 = case shown="True" w250 {
          frame False {
          }
          frame True {
            w255 = FALSE ("Ack hard alarm!")
            n130 = property on="System Alarm" class="Bool (strict)"("Value"=w255) -> ()  [unwired: 2 in, 2 out]
            n131 = property on="Hard Alarm" class="Bool (strict)"("Value"=w255) -> ()  [unwired: 2 in, 2 out]
          }
        }
        n132 = case shown="False" "Acknowledge" {
          tunnel: [w253 0.0 ("Numeric")] -> w247
          tunnel: w248 -> [w253 _]
          frame False {
          }
          frame True {
          }
        }
      }
      frame True {
        n133 = local read "Table"() -> (w262:string[][])
        n134 = call "Error list.vi"("Error code"=w259, "Error array in"=w262) -> ("Hard alarm?"=w256:bool, "Error array out"=w261:string[][])  [unwired: 8 in]
        "Hard Alarm" <- w256
        "System Alarm" <- w256
        n135 = Not(x=w256) -> (.not. x?=w257:bool)
        "Soft Alarm" <- w257
        n136 = case shown="True" w257 {
          frame False {
          }
          frame True {
            n137 = property on="Alarm ack" class="Bool"("DisabledEnum"=T13."Enabled" ("Disabled")) -> ()  [unwired: 2 in, 2 out]
          }
        }
        n138 = local write "Table"(w261) -> ()
        n139 = local write "Acknowledge"(FALSE ("Acknowledge")) -> ()
        n140 = property on="Tab Control" class="TabCtl (strict)"("Value"=6) -> ()  [unwired: 2 in, 2 out]
      }
    }
    n141 = local read "Full system?"() -> (w105:bool)
    n142 = Index Array(array=w43, index #1=0 ("index"), index #2=1 ("index"), index #3=2 ("index"), index #4=3 ("index"), index #5=4 ("index"), index #6=5 ("index"), index #7=7 ("index"), index #8=8 ("index"), index #9=9 ("index"), index #10=10 ("index"), index #11=12 ("index"), index #12=13 ("index"), index #13=14 ("index"), index #14=15 ("index"), index #15=16 ("index"), index #16=17 ("index"), index #17=32 ("index"), index #18=33 ("index"), index #19=34 ("index"), index #20=35 ("index"), index #21=36 ("index"), index #22=38 ("index"), index #23=39 ("index"), index #24=40 ("index"), index #25=41 ("index"), index #26=42 ("index"), index #27=43 ("index"), index #28=44 ("index"), index #29=45 ("index"), index #30=46 ("index"), index #31=47 ("index")) -> (element #1=w102:dbl, element #2=w101:dbl, element #3=w98:dbl, element #4=w96:dbl, element #5=w97:dbl, element #6=w95:dbl, element #7=w94:dbl, element #8=w93:dbl, element #9=w92:dbl, element #10=w91:dbl, element #11=w86:dbl, element #12=w85:dbl, element #13=w84:dbl, element #14=w83:dbl, element #15=w82:dbl, element #16=w81:dbl, element #17=w75:dbl, element #18=w74:dbl, element #19=w73:dbl, element #20=w72:dbl, element #21=w71:dbl, element #22=w66:dbl, element #23=w65:dbl, element #24=w64:dbl, element #25=w63:dbl, element #26=→"Furnace temp 1":dbl, element #27=→"Furnace temp 2":dbl, element #28=w56:dbl, element #29=w55:dbl, element #30=w52:dbl, element #31=w51:dbl)
    n143 = Build Array(w105, w104) -> (w106:bool[])
    n144 = Boolean Array To Number(Boolean array=w106) -> (number=w103:u32)
    n145 = case shown="3" w103 {
      tunnel: w102 -> [w200 w202 _ _]
      tunnel: w101 -> [_ w201 _ _]
      tunnel: [w200 w202 w203 w204] -> w100
      tunnel: [0.0 ("y") w201 w203 w204] -> w99
      frame 0, Default {
      }
      frame 1 {
      }
      frame 2 {
        w203 = 0.0 ("y")
      }
      frame 3 {
        w204 = 0.0 ("y")
      }
    }
    n146 = Merge Signals(w86, w85, w84, w83, w82, w81) -> (→"Sample Temperatures (°C)":dynamicdata)
    n147 = Merge Signals(w75, w74, w73, w72, w71) -> (→"System Temperatures (°C)":dynamicdata)
    n148 = Merge Signals(w56, w52) -> (→"NO Concentration (ppm)":dynamicdata)
    n149 = Merge Signals(w55, w51, w44) -> (→"Lambda":dynamicdata)
    n150 = Merge Signals(w66, w65, w64, w63) -> (→"Heat Exchanger Temperatures (°C)":dynamicdata)
    n151 = Merge Signals(w100, w99) -> (→"Flow Rate (g/s)":dynamicdata)
    n152 = Merge Signals(w98, w96, w95, w94, w93, w91) -> (→"M584L Upstream & Downstream":dynamicdata)
    n153 = Merge Signals(w97, w92) -> (→"HC Concentration (ppm)":dynamicdata)
    n154 = local read "stop 2"() -> (w167:bool)
    n155 = node-c288() -> ()  [unwired: 1 in, 1 out]
  }
  n156 = while {
    tunnel: w35 -> [w329]
    tunnel: w19 -> [w327]
    tunnel: w21 -> [w326]
    tunnel: [FALSE ("stop 2")] -> w9
    stop <- w330 stop-if-true
    n157 = Dequeue Element(queue=w329) -> (element=w328:T10)  [unwired: 2 in, 3 out]
    n158 = case shown="\"main\", Default" w328 {
      tunnel: w327 -> [_ _ _ w375 w386 w422 w456 _ _ _ _ _ _ _ w819 _ _ _ _ _ _ _]
      tunnel: w326 -> [_ _ _ _ _ _ _ _ w469 w484 w539 w584 _ _ _ _ _ _ _ _ _ _]
      frame "main", Default {
        # "0 NOx Conc\n1 CO conc %\n2 HC conc %\n3 Bleed H2O \n4 Bleed CO2\n5 Bleed N2 \n6 lambda P\n7 lambda I\n8 lambda D\n9 purge duration\n10 Target furnace lambda\n11 HC reaction ct\n12 Full system\n13 Log interval"
        n159 = local read "output cluster"() -> (w349:T2)
        n160 = Unbundle(w349) -> ("NOx Concentration (ppm)"=w335:T1, "CO concentration %"=w334:T1, "HC concentration %"=w333:T1, "Bleed H2O %"=w332:T1, "Bleed CO2 %"=w331:T1, "Bleed N2 %"=w346:T1, "lambda P"=w345:T1, "lambda I"=w344:T1, "lambda D"=w347:T1, "Purge duration (seconds)"=w348:T1, "Target furnace lambda"=w340:T1, "HC reaction constant"=w339:T1, w341:i16, "Log interval (HRS)"=→"Log interval (seconds)":T1)
        n161 = local read "Test Flow Rate(g/s)"() -> (w361:T1)
        n162 = local read "Test number"() -> (w366:u16)
        n163 = local read "Connected?"() -> (w355:bool)
        n164 = local read "NO ppm Loff"() -> (w351:T1)
        n165 = local read "NO:CO Ratio"() -> (w350:T1)
        n166 = local read "Inlet LAMBDA"() -> (w353:T1)
        n167 = local read "Inlet O2 (%)"() -> (w352:T1)
        n168 = Boolean To (0,1)(Boolean=w355) -> (0, 1=w338:i16)
        n169 = Not Equal To 0?(x=w341) -> (x != 0?=→"Full system?":bool)
        n170 = Build Array("Stop Cmd", w366, w361, "Test Start Temperature (°C)", "Test Stop temperature (°C)", "Furnace Ramp Rate (°C/min)", w353, w352, "Inlet LAMBDA Rich", "Inlet LAMBDA Lean", "Inlet Temperature (°C)", "NO ppm SW", w351, w350, "Temperature Limit (°C)", w338, "Inlet temp Age", "Flow rate Age", w335, w334, w333, w332, w331, w346, w345, w344, w347, w348, w340, w339, w341) -> (w357:T1[])
        n171 = shared-variable "NI-cRIO9074-018C1D8D\\Library 1.lvlib\\Control Variables"(w357) -> ()  [unwired: 1 in, 1 out]
      }
      frame "start test" {
        w367 = FALSE
        n172 = property on="Pass" class="Bool (strict)"("Value"=w367) -> ()  [unwired: 2 in, 2 out]
        n173 = property on="Fail" class="Bool (strict)"("Value"=w367) -> ()  [unwired: 2 in, 2 out]
        n174 = local write "Pass"(w367) -> ()
        n175 = local write "Fail"(w367) -> ()
        n176 = shared-variable "NI-cRIO9074-018C1D8D\\Library 1.lvlib\\Enum 1"("Enum 1") -> ()  [unwired: 1 in, 1 out]
      }
      frame "clear table 1" {
        n177 = property on="Sub-Cycle Name" class="Str"("Value"="" ("Subcycle name")) -> ()  [unwired: 2 in, 2 out]
        n178 = local write "Flag1"(FALSE) -> ()
        n179 = local write "Sub-Cycle Pattern"(string[][] [["", "0", "", "", "", "", "", "", "", "", "", "", ""], ["", "", "", "", "", "", "", "", "", "", "", "", ""], ["", "", "", "", "", "", "", "", "", "", "", "", ""], ["", "", "", "", "", "", "", "", "", "", "", "", ""], ["", "", "", "", "", "", "", "", "", "", "", "", ""], ["", "", "", "", "", "", "", "", "", "", "", "", ""], ["", "", "", "", "", "", "", "", "", "", "", "", ""], ["", "", "", "", "", "", "", "", "", "", "", "", ""], ["", "", "", "", "", "", "", "", "", "", "", "", ""], ["", "", "", "", "", "", "", "", "", "", "", "", ""], ["", "", "", "", "", "", "", "", "", "", "", "", ""], ["", "", "", "", "", "", "", "", "", "", "", "", ""], ["", "", "", "", "", "", "", "", "", "", "", "", ""], ["", "", "", "", "", "", "", "", "", "", "", "", ""], ["", "", "", "", "", "", "", "", "", "", "", "", ""], ["", "", "", "", "", "", "", "", "", "", "", "", ""], ["", "", "", "", "", "", "", "", "", "", "", "", ""], ["", "", "", "", "", "", "", "", "", "", "", "", ""], ["", "", "", "", "", "", "", "", "", "", "", "", ""], ["", "", "", "", "", "", "", "", "", "", "", "", ""], ["", "", "", "", "", "", "", "", "", "", "", "", ""], ["", "", "", "", "", "", "", "", "", "", "", "", ""], ["", "", "", "", "", "", "", "", "", "", "", "", ""], ["", "", "", "", "", "", "", "", "", "", "", "", ""], ["", "", "", "", "", "", "", "", "", "", "", "", ""], ["", "", "", "", "", "", "", "", "", "", "", "", ""], ["", "", "", "", "", "", "", "", "", "", "", "", ""], ["", "", "", "", "", "", "", "", "", "", "", "", ""], ["", "", "", "", "", "", "", "", "", "", "", "", ""], ["", "", "", "", "", "", "", "", "", "", "", "", ""], ["", "", "", "", "", "", "", "", "", "", "", "", ""]]) -> ()
      }
      frame "update list 1" {
        n180 = String To Path(string=w375) -> (path=w374:path)
        n181 = List Folder(path=w374, pattern="*.eyes") -> (filenames=w373:string[])  [unwired: 2 in, 3 out]
        n182 = property on="Sub-Cycle List" class="LstBox (strict)"("Item Names"=w373) -> ()  [unwired: 2 in, 2 out]
      }
      frame "save subc" {
        w379 = ".eyes" ("string")
        n183 = local read "Sub-Cycle Name"() -> (w378:T5)
        n184 = String To Path(string=w386) -> (path=w391:path)
        n185 = Equal?(x=w378, y="") -> (x = y?=w383:bool)
        n186 = List Folder(path=w391, pattern="*.eyes" ("string")) -> (filenames=w390:string[])  [unwired: 2 in, 3 out]
        n187 = Concatenate Strings(w378, w379) -> (w377:string)
        n188 = Concatenate Strings(w386, w378, w379) -> (w392:string)
        n189 = Search 1D Array(1D array=w390, element=w377) -> (index of element=w389:i32)  [unwired: 1 in]
        n190 = case shown="True" w383 {
          tunnel: [TRUE FALSE] -> w382
          frame False {
          }
          frame True {
            n191 = One Button Dialog(message="Insert file name!") -> ()  [unwired: 1 in, 1 out]
          }
        }
        n192 = String To Path(string=w392) -> (path=w385:path)
        n193 = Equal?(x=w389, y=-1) -> (x = y?=w387:bool)
        n194 = case shown="False" w387 {
          selector: w387 -> [_ w398]
          tunnel: [w396 w398] -> w381
          frame False {
            n195 = Two Button Dialog(message="A file with this name already exists!\nDo you want to overwrite?") -> (T button?=w396:bool)  [unwired: 2 in]
          }
          frame True {
          }
        }
        n196 = And(x=w381, y=w382) -> (x .and. y?=w380:bool)
        n197 = case shown="True" w380 {
          tunnel: w385 -> [_ w403]
          frame False {
          }
          frame True {
            n198 = local read "Sub-Cycle Pattern"() -> (w402:string[][])
            n199 = call "Table check.vi"("Input table"=w402) -> ("Incomplete?"=w400:bool, "Length"=w401:i32)  [unwired: 9 in]
            n200 = case shown="False" w400 {
              tunnel: w402 -> [w411 _]
              tunnel: w403 -> [w410 _]
              tunnel: w401 -> [w409 _]
              tunnel: string[] [] -> [w408 _]
              frame False {
                n201 = for {
                  N: w409 -> [_]
                  tunnel: w411 -> [w418]
                  shift-right: [w415] -> w407
                  shift-left: w408 -> [w416]
                  i -> [w417]
                  n202 = Index Array(array=w418, index (row)=w417) -> (element=w414:string[])  [unwired: 1 in]
                  n203 = Delete From Array(array=w414, index=0) -> (array with subset deleted=w413:string[])  [unwired: 1 in, 1 out]
                  n204 = Build Array (concatenate)(w416, w413) -> (w415:string[])
                }
                n205 = Build Array (concatenate)("SubCycle Data File for EYECAT - do not modify", w407) -> (w405:string[])
                n206 = call-poly <vilib>:"Write To Spreadsheet File.vi"("1D data"=w405, "file path (dialog if empty)"=w410) -> ()  [unwired: 6 in, 1 out]
              }
              frame True {
                n207 = One Button Dialog(message="The table is incomplete!\nplease review and save again!") -> ()  [unwired: 1 in, 1 out]
              }
            }
            n208 = local write "Flag1"(FALSE) -> ()
          }
        }
      }
      frame "load subc" {
        n209 = local read "Flag1"() -> (w423:bool)
        n210 = case shown="True" w423 {
          tunnel: [w450 w452] -> w421
          tunnel: w422 -> [w450 w452]
          tunnel: [TRUE w451] -> w420
          frame False {
          }
          frame True {
            n211 = Two Button Dialog(message="The table has been modified.\nDo you want to continue?") -> (T button?=w451:bool)  [unwired: 2 in]
          }
        }
        n212 = case shown="True" w420 {
          tunnel: w421 -> [_ w427]
          frame False {
          }
          frame True {
            n213 = property on="Sub-Cycle List" class="LstBox (strict)"() -> ("Item Names"=w439:string[])  [unwired: 2 in, 2 out]
            n214 = Index Array(array=w439, index="Sub-Cycle List") -> (element=w426:string)
            n215 = Concatenate Strings(w427, w426) -> (w437:string)
            n216 = Search/Split String(string=w426, search string/char (-)=".") -> (substring before match=w424:string)  [unwired: 1 in, 2 out]
            n217 = local write "Sub-Cycle Name"(w424) -> ()
            n218 = String To Path(string=w437) -> (path=w436:path)
            n219 = call-poly <vilib>:"Read From Spreadsheet File.vi"("file path (dialog if empty)"=w436) -> ("first row"=w432:string[])  [unwired: 6 in, 4 out]
            n220 = Delete From Array(array=w432, length=1, index=0) -> (array with subset deleted=w429:string[])  [unwired: 1 out]
            n221 = Array Size(array=w429) -> (size(s)=w435:i32)
            n222 = Divide(x=w435, y=12) -> (x/y=w428:dbl)
            n223 = for {
              N: w428 -> [_]
              shift-right: [w445] -> _
              shift-left: w429 -> [w448]
              tunnel: [w444] -> w433 mode=indexing
              i -> [w443]
              n224 = Increment(x=w443) -> (x+1=w442:i32)
              n225 = Delete From Array(array=w448, length=12, index=0) -> (deleted portion=w440:string[], array with subset deleted=w445:string[])
              n226 = Number To Decimal String(number=w442) -> (decimal integer string=w441:string)  [unwired: 1 in]
              n227 = Build Array (concatenate)(w441, w440) -> (w444:string[])
            }
            n228 = local write "Sub-Cycle Pattern"(w433) -> ()
          }
        }
      }
      frame "delete subc" {
        n229 = Two Button Dialog(message="This operation will permanently delete this file!\nDo you want to continue?") -> (T button?=w455:bool)  [unwired: 2 in]
        n230 = case shown="True" w455 {
          tunnel: w456 -> [_ w461]
          frame False {
          }
          frame True {
            n231 = local read "Sub-Cycle List"() -> (w458:i32)
            n232 = property on="Sub-Cycle List" class="LstBox (strict)"() -> ("Item Names"=w459:string[])  [unwired: 2 in, 2 out]
            n233 = Index Array(array=w459, index=w458) -> (element=w463:string)
            n234 = Concatenate Strings(w461, w463) -> (w462:string)
            n235 = local write "Flag1"(FALSE) -> ()
            n236 = String To Path(string=w462) -> (path=w460:path)
            n237 = Delete(path (use dialog)=w460) -> ()  [unwired: 4 in, 3 out]
          }
        }
      }
      frame "clear table 2" {
        n238 = property on="Cycle Name" class="Str"("Value"="" ("Subcycle name")) -> ()  [unwired: 2 in, 2 out]
        n239 = local write "Flag 2"(FALSE) -> ()
        n240 = local write "Cycle Pattern"(string[][] [["", "", "", "", ""], ["", "", "", "", ""], ["", "", "", "", ""], ["", "", "", "", ""], ["", "", "", "", ""], ["", "", "", "", ""], ["", "", "", "", ""], ["", "", "", "", ""], ["", "", "", "", ""], ["", "", "", "", ""], ["", "", "", "", ""], ["", "", "", "", ""], ["", "", "", "", ""], ["", "", "", "", ""], ["", "", "", "", ""], ["", "", "", "", ""], ["", "", "", "", ""], ["", "", "", "", ""], ["", "", "", "", ""], ["", "", "", "", ""], ["", "", "", "", ""], ["", "", "", "", ""], ["", "", "", "", ""], ["", "", "", "", ""], ["", "", "", "", ""], ["", "", "", "", ""], ["", "", "", "", ""], ["", "", "", "", ""], ["", "", "", "", ""], ["", "", "", "", ""], ["", "", "", "", ""]]) -> ()
      }
      frame "update list 2" {
        n241 = String To Path(string=w469) -> (path=w470:path)
        n242 = List Folder(path=w470, pattern="*.eyec") -> (filenames=w468:string[])  [unwired: 2 in, 3 out]
        n243 = property on="Cycle List" class="LstBox (strict)"("Item Names"=w468) -> ()  [unwired: 2 in, 2 out]
      }
      frame "save cycle" {
        w471 = ".eyec" ("string")
        n244 = local read "Cycle Name"() -> (w472:T5)
        n245 = String To Path(string=w484) -> (path=w485:path)
        n246 = List Folder(path=w485, pattern="*.eyec" ("string")) -> (filenames=w483:string[])  [unwired: 2 in, 3 out]
        n247 = Equal?(x=w472, y="") -> (x = y?=w478:bool)
        n248 = Concatenate Strings(w472, w471) -> (w474:string)
        n249 = Search 1D Array(1D array=w483, element=w474) -> (index of element=w482:i32)  [unwired: 1 in]
        n250 = Concatenate Strings(w484, w472, w471) -> (w487:string)
        n251 = case shown="True" w478 {
          tunnel: [TRUE FALSE] -> w476
          frame False {
          }
          frame True {
            n252 = One Button Dialog(message="Insert file name!") -> ()  [unwired: 1 in, 1 out]
          }
        }
        n253 = String To Path(string=w487) -> (path=w486:path)
        n254 = Equal?(x=w482, y=-1) -> (x = y?=w480:bool)
        n255 = case shown="False" w480 {
          selector: w480 -> [_ w536]
          tunnel: [w534 w536] -> w477
          frame False {
            n256 = Two Button Dialog(message="A file with this name already exists!\nDo you want to overwrite?") -> (T button?=w534:bool)  [unwired: 2 in]
          }
          frame True {
          }
        }
        n257 = And(x=w477, y=w476) -> (x .and. y?=w475:bool)
        n258 = case shown="True" w475 {
          tunnel: w486 -> [_ w494]
          frame False {
          }
          frame True {
            n259 = local read "Cycle Pattern"() -> (w493:string[][])
            n260 = call "Table check.vi"("Input table"=w493) -> ("Incomplete?"=w491:bool, "Length"=w492:i32)  [unwired: 9 in]
            n261 = case shown="False" w491 {
              tunnel: w494 -> [w503 _]
              tunnel: w493 -> [w502 _]
              tunnel: w492 -> [w495 _]
              frame False {
                n262 = Number To Decimal String(number=w495) -> (decimal integer string=w498:string)  [unwired: 1 in]
                n263 = for {
                  N: w495 -> [_]
                  tunnel: w502 -> [w532]
                  shift-right: [w520] -> w499
                  shift-left: string[] [] -> [w530]
                  i -> [w531]
                  w511 = 12 ("length")
                  n264 = Index Array(array=w532, index (row)=w531) -> (element=w526:string[])  [unwired: 1 in]
                  n265 = Index Array(array=w526, index=3) -> (element=w516:string)
                  n266 = Index Array(array=w526, index=1) -> (element=w515:string)
                  n267 = Concatenate Strings("C:\\Setup Files\\Subcycles Folder\\", w515) -> (w527:string)
                  n268 = String To Path(string=w527) -> (path=w528:path)
                  n269 = call-poly <vilib>:"Read From Spreadsheet File.vi"("file path (dialog if empty)"=w528) -> ("first row"=w519:string[])  [unwired: 6 in, 4 out]
                  n270 = Delete From Array(array=w519, length=1, index=0) -> (array with subset deleted=w513:string[])  [unwired: 1 out]
                  n271 = String Length(string=w513) -> (length=w522:i32[])
                  n272 = Array Size(array=w522) -> (size(s)=w514:i32)
                  n273 = Divide(x=w514, y=w511) -> (x/y=w512:dbl)
                  n274 = Decrement(x=w512) -> (x-1=w504:dbl)
                  n275 = Multiply(x=w511, y=w504) -> (x*y=w510:dbl)
                  n276 = Number To Decimal String(number=w504) -> (decimal integer string=w521:string)  [unwired: 1 in]
                  n277 = Delete From Array(array=w513, length=12, index=w510) -> (deleted portion=w507:string[], array with subset deleted=w508:string[])
                  n278 = Index Array(array=w507, index=0) -> (element=w505:string)
                  n279 = Build Array (concatenate)(w515, w516, w521, w505, w508) -> (w525:string[])
                  n280 = Build Array (concatenate)(w530, w525) -> (w520:string[])
                }
                n281 = local write "Flag 2"(FALSE) -> ()
                n282 = Build Array (concatenate)("Cycle Data File for EYECAT - do not modify", w498, w499) -> (w500:string[])
                n283 = call-poly <vilib>:"Write To Spreadsheet File.vi"("1D data"=w500, "file path (dialog if empty)"=w503) -> ()  [unwired: 6 in, 1 out]
              }
              frame True {
                n284 = One Button Dialog(message="The table is incomplete!\nplease review and save again!") -> ()  [unwired: 1 in, 1 out]
              }
            }
          }
        }
      }
      frame "load cycle" {
        n285 = local read "Flag 2"() -> (w540:bool)
        n286 = case shown="True" w540 {
          tunnel: [w579 w581] -> w537
          tunnel: w539 -> [w579 w581]
          tunnel: [TRUE ("T button?") w580] -> w538
          frame False {
          }
          frame True {
            n287 = Two Button Dialog(message="The table has been modified.\nDo you want to continue?") -> (T button?=w580:bool)  [unwired: 2 in]
          }
        }
        n288 = case shown="True" w538 {
          tunnel: w537 -> [_ w543]
          frame False {
          }
          frame True {
            n289 = property on="Cycle List" class="LstBox (strict)"() -> ("Item Names"=w559:string[])  [unwired: 2 in, 2 out]
            n290 = Index Array(array=w559, index="Cycle List") -> (element=w545:string)
            n291 = Concatenate Strings(w543, w545) -> (w558:string)
            n292 = Search/Split String(string=w545, search string/char (-)=".") -> (substring before match=w544:string)  [unwired: 1 in, 2 out]
            n293 = String To Path(string=w558) -> (path=w557:path)
            n294 = local write "Cycle Name"(w544) -> ()
            n295 = call-poly <vilib>:"Read From Spreadsheet File.vi"("file path (dialog if empty)"=w557) -> ("first row"=w541:string[])  [unwired: 6 in, 4 out]
            n296 = Delete From Array(array=w541, length=2, index=0) -> (array with subset deleted=w542:string[])  [unwired: 1 out]
            n297 = Index Array(array=w541, index=1) -> (element=w556:string)
            n298 = Decimal String To Number(string=w556) -> (number=w555:i32)  [unwired: 2 in, 1 out]
            n299 = for {
              N: w555 -> [_]
              tunnel: w542 -> [w577]
              tunnel: [w572] -> w550 mode=indexing
              shift-right: [w562] -> _
              shift-left: 0 ("x") -> [w563]
              i -> [w576]
              w573 = ""
              n300 = Increment(x=w563) -> (x+1=w561:i32)
              n301 = Increment(x=w561) -> (x+1=w569:i32)
              n302 = Increment(x=w576) -> (x+1=w571:i32)
              n303 = Number To Decimal String(number=w571) -> (decimal integer string=w570:string)  [unwired: 1 in]
              n304 = Index Array(array=w577, index #1=w563, index #2=w561, index #3=w569) -> (element #1=w575:string, element #2=w574:string, element #3=w568:string)
              n305 = Build Array(w570, w575, w573, w574, w573) -> (w572:string[])
              n306 = Decimal String To Number(string=w568) -> (number=w567:i32)  [unwired: 2 in, 1 out]
              n307 = Multiply(x=w567, y=12 ("x")) -> (x*y=w565:i32)
              n308 = Compound Arithmetic op=ADD(w565, 4, w563) -> (w562:i32)
            }
            n309 = Insert Into Array(array=string[][] [["", "", "", "", ""], ["", "", "", "", ""], ["", "", "", "", ""], ["", "", "", "", ""], ["", "", "", "", ""], ["", "", "", "", ""], ["", "", "", "", ""], ["", "", "", "", ""], ["", "", "", "", ""], ["", "", "", "", ""], ["", "", "", "", ""], ["", "", "", "", ""], ["", "", "", "", ""], ["", "", "", "", ""], ["", "", "", "", ""], ["", "", "", "", ""], ["", "", "", "", ""], ["", "", "", "", ""], ["", "", "", "", ""], ["", "", "", "", ""], ["", "", "", "", ""], ["", "", "", "", ""], ["", "", "", "", ""], ["", "", "", "", ""], ["", "", "", "", ""], ["", "", "", "", ""], ["", "", "", "", ""], ["", "", "", "", ""], ["", "", "", "", ""], ["", "", "", "", ""], ["", "", "", "", ""]], index (row)=0, new element=w550) -> (w549:string[][])  [unwired: 1 in]
            n310 = local write "Cycle Pattern"(w549) -> ()
          }
        }
      }
      frame "delete cycle" {
        n311 = Two Button Dialog(message="This operation will permanently delete this file!\nDo you want to continue?") -> (T button?=w585:bool)  [unwired: 2 in]
        n312 = case shown="True" w585 {
          tunnel: w584 -> [_ w590]
          frame False {
          }
          frame True {
            n313 = local read "Cycle List"() -> (w591:i32)
            n314 = property on="Cycle List" class="LstBox (strict)"() -> ("Item Names"=w592:string[])  [unwired: 2 in, 2 out]
            n315 = Index Array(array=w592, index=w591) -> (element=w589:string)
            n316 = Concatenate Strings(w590, w589) -> (w588:string)
            n317 = String To Path(string=w588) -> (path=w587:path)
            n318 = Delete(path (use dialog)=w587) -> ()  [unwired: 4 in, 3 out]
            n319 = local write "Flag 2"(FALSE) -> ()
          }
        }
      }
      frame "calc HC CO" {
        n320 = local read "Sub-Cycle Pattern"() -> (w609:string[][])
        n321 = Index Array(array=w609, index (col) #1=3 ("disabled index (col)"), index (col) #2=4 ("index (col)"), index (col) #3=11 ("index (col)")) -> (element #1=w599:string[], element #2=w606:string[], element #3=w593:string[])  [unwired: 3 in]
        n322 = Array Size(array=w599) -> (size(s)=w597:i32)
        n323 = Search 1D Array(1D array=w599, element="") -> (index of element=w596:i32)  [unwired: 1 in]
        n324 = Equal?(x=w596, y=-1) -> (x = y?=w598:bool)
        n325 = Select(t=w597, s=w598, f=w596) -> (s? t:f=w595:i32)
        n326 = for {
          N: w595 -> [_]
          tunnel: [w620] -> w603 mode=indexing
          tunnel: [w619] -> w602 mode=indexing
          tunnel: w599 -> [w618] mode=indexing
          tunnel: w606 -> [w617] mode=indexing
          tunnel: w593 -> [w616] mode=indexing
          w615 = ""
          n327 = Not Equal?(x=w618, y=w615) -> (x != y?=w614:bool)
          n328 = Not Equal?(x=w617, y=w615) -> (x != y?=w613:bool)
          n329 = Not Equal?(x=w616, y=w615) -> (x != y?=w612:bool)
          n330 = Compound Arithmetic op=AND(w614, w613, w612) -> (w611:bool)
          n331 = case shown="True" w611 {
            tunnel: w618 -> [_ w649]
            tunnel: w617 -> [_ w648]
            tunnel: [w621 w645] -> w619
            tunnel: [w621 w644] -> w620
            tunnel: w616 -> [_ w622]
            frame False {
              w621 = ""
            }
            frame True {
              # "O2Eq"
              n332 = Fract/Exp String To Number(string=w622) -> (number=w623:dbl)  [unwired: 3 in, 1 out]
              n333 = Fract/Exp String To Number(string=w649) -> (number=w630:dbl)  [unwired: 3 in, 1 out]
              n334 = Fract/Exp String To Number(string=w648) -> (number=w626:dbl)  [unwired: 3 in, 1 out]
              n335 = Decrement(x=w630) -> (x-1=w631:dbl)
              n336 = Divide(x=w623, y=20000.0) -> (x/y=w624:dbl)
              n337 = Multiply(x=4.76, y=w630) -> (x*y=w635:dbl)
              n338 = Multiply(x=w631, y=100.0) -> (x*y=w633:dbl)
              n339 = Add(x=w626, y=w624) -> (x+y=w627:dbl)
              n340 = Add(x=0.33, y=w635) -> (x+y=w637:dbl)
              n341 = Divide(x=w633, y=w637) -> (x/y=w638:dbl)
              n342 = Subtract(x=w627, y=w638) -> (x-y=w640:dbl)
              n343 = Multiply(x=w640, y=2.0) -> (x*y=w628:dbl)
              n344 = Divide(x=w640, y=5.0) -> (x/y=w629:dbl)
              n345 = Number To Fractional String(number=w629, width (-)=i16 6, precision (6)=i16 3) -> (F-format string=w644:string)  [unwired: 1 in]
              n346 = Number To Fractional String(number=w628, width (-)=i16 6, precision (6)=i16 2) -> (F-format string=w645:string)  [unwired: 1 in]
            }
          }
        }
        n347 = Replace Array Subset(array=w609, new element #1=w603, index (col) #1=5 ("disabled index (col)"), new element #2=w602, index (col) #2=6 ("disabled index (col)")) -> (w607:string[][])  [unwired: 2 in]
        n348 = local write "Sub-Cycle Pattern"(w607) -> ()
      }
      frame "Total time calc" {
        w664 = i16 2 ("width (-)")
        w671 = ":"
        n349 = local read "Cycle Pattern"() -> (w678:string[][])
        n350 = Index Array(array=w678, index (col)=4 ("disabled index (col)")) -> (element=w651:string[])  [unwired: 1 in]
        n351 = Array Size(array=w651) -> (size(s)=w653:i32)
        n352 = Search 1D Array(1D array=w651, element="") -> (index of element=w652:i32)  [unwired: 1 in]
        n353 = Equal?(x=w652, y=-1) -> (x = y?=w654:bool)
        n354 = Select(t=w653, s=w654, f=w652) -> (s? t:f=w650:i32)
        n355 = for {
          N: w650 -> [_]
          tunnel: w651 -> [w686] mode=indexing
          shift-right: [w688] -> w674
          shift-left: 0 -> [w689]
          n356 = xnode "Match Regular Expression"("input string"=w686, "regular expression"=":" ("search string/char (-)")) -> ("before match"=w685:string, "after match"=w682:string)  [unwired: 4 in, 3 out]
          n357 = Decimal String To Number(string=w685) -> (number=w684:i32)  [unwired: 2 in, 1 out]
          n358 = Decimal String To Number(string=w682) -> (number=w681:i32)  [unwired: 2 in, 1 out]
          n359 = Multiply(x=w684, y=60) -> (x*y=w680:i32)
          n360 = Add(x=w680, y=w681) -> (x+y=w679:i32)
          n361 = Add(x=w679, y=w689) -> (x+y=w688:i32)
        }
        n362 = local read "Total Number of Cycles"() -> (w675:T1)
        n363 = Multiply(x=w674, y=w675) -> (x*y=w670:T1)
        n364 = Quotient & Remainder(x=w670, y=3600.0) -> (x-y*floor(x/y)=w657:T1, floor(x/y)=w667:T1)
        n365 = Quotient & Remainder(x=w657, y=60.0) -> (x-y*floor(x/y)=w665:T1, floor(x/y)=w666:T1)
        n366 = Number To Decimal String(number=w667) -> (decimal integer string=w672:string)  [unwired: 1 in]
        n367 = Number To Decimal String(number=w666, width (-)=w664) -> (decimal integer string=w668:string)
        n368 = Number To Decimal String(number=w665, width (-)=w664) -> (decimal integer string=w663:string)
        n369 = Concatenate Strings(w672, w671, w668, w671, w663) -> (w662:string)
        n370 = call <vilib>:"Search and Replace Pattern.vi"("string"=w662, "regular expression (\"\")"=" " ("replace string (\"\")"), "replace string (\"\")"="0" ("replace string (\"\")"), "replace all? (F)"=TRUE) -> ("result string"=→"Total Test Duration (hrs)":string)  [unwired: 1 in, 1 out]
      }
      frame "update Cycle pattern " {
        n371 = local read "Cycle Pattern"() -> (w817:string[][])
        n372 = Index Array(array=w817, index (col)=1 ("disabled index (col)")) -> (element=w802:string[])  [unwired: 1 in]
        n373 = String To Path(string=w819) -> (path=w820:path)
        n374 = Array Size(array=w802) -> (size(s)=w805:i32)
        n375 = Search 1D Array(1D array=w802, element="") -> (index of element=w804:i32)  [unwired: 1 in]
        n376 = List Folder(path=w820, pattern="*.eyes") -> (filenames=w818:string[])  [unwired: 2 in, 3 out]
        n377 = Equal?(x=w804, y=-1) -> (x = y?=w806:bool)
        n378 = Select(t=w805, s=w806, f=w804) -> (s? t:f=w803:i32)
        n379 = for {
          N: w803 -> [_]
          tunnel: w817 -> [w836] mode=indexing
          tunnel: w819 -> [w829]
          tunnel: [w831] -> w812 mode=indexing
          tunnel: [w833] -> w816 mode=indexing
          tunnel: [w830] -> w813 mode=indexing
          tunnel: w818 -> [w828]
          tunnel: [w823] -> w809 mode=indexing
          n380 = Index Array(array=w836, index #1=1 ("index"), index #2=3 ("index")) -> (element #1=w827:string, element #2=w832:string)
          n381 = Search 1D Array(1D array=w828, element=w827) -> (index of element=w826:i32)  [unwired: 1 in]
          n382 = Not Equal?(x=w826, y=-1) -> (x != y?=w824:bool)
          n383 = case shown="True" w824 {
            tunnel: [w840 w854] -> w833
            tunnel: w832 -> [_ w850]
            tunnel: [w840 w848] -> w831
            tunnel: [w840 w847] -> w830
            tunnel: w829 -> [_ w846]
            tunnel: w827 -> [w839 w845]
            tunnel: [w838 w845] -> w823
            frame False {
              w840 = "N/A" ("String")
              n384 = Concatenate Strings(w839, " - File NOT AVAILABLE !!!" ("string")) -> (w838:string)
            }
            frame True {
              w858 = i16 2 ("width (-)")
              n385 = Concatenate Strings(w846, w845) -> (w876:string)
              n386 = String To Path(string=w876) -> (path=w875:path)
              n387 = call <vilib>:"Search and Replace Pattern.vi"("string"=w850, "regular expression (\"\")"="[a-x ]" ("format string"), "replace string (\"\")"="", "replace all? (F)"=TRUE) -> ("result string"=w847:string)  [unwired: 1 in, 1 out]
              n388 = call-poly <vilib>:"Read From Spreadsheet File.vi"("file path (dialog if empty)"=w875) -> ("first row"=w844:string[])  [unwired: 6 in, 4 out]
              n389 = Delete From Array(array=w844, length=1, index=0) -> (array with subset deleted=w843:string[])  [unwired: 1 out]
              n390 = Array Size(array=w843) -> (size(s)=w874:i32)
              n391 = Equal?(x=w847, y="") -> (x = y?=w862:bool)
              n392 = Subtract(x=w874, y=12) -> (x-y=w872:i32)
              n393 = Select(t="0", s=w862, f=w847) -> (s? t:f=w861:string)
              n394 = Index Array(array=w843, index=w872) -> (element=w848:string)
              n395 = Decimal String To Number(string=w861) -> (number=w871:i32)  [unwired: 2 in, 1 out]
              n396 = Decimal String To Number(string=w848) -> (number=w870:i32)  [unwired: 2 in, 1 out]
              n397 = Multiply(x=w871, y=w870) -> (x*y=w869:i32)
              n398 = Quotient & Remainder(x=w869, y=60) -> (x-y*floor(x/y)=w867:i32, floor(x/y)=w866:i32)
              n399 = Number To Decimal String(number=w867, width (-)=w858) -> (decimal integer string=w864:string)
              n400 = Number To Decimal String(number=w866, width (-)=w858) -> (decimal integer string=w863:string)
              n401 = Concatenate Strings(w863, ":", w864) -> (w857:string)
              n402 = call <vilib>:"Search and Replace Pattern.vi"("string"=w857, "regular expression (\"\")"=" " ("replace string (\"\")"), "replace string (\"\")"="0" ("replace string (\"\")"), "replace all? (F)"=TRUE) -> ("result string"=w854:string)  [unwired: 1 in, 1 out]
            }
          }
        }
        n403 = Replace Array Subset(array=w817, new element #1=w809, index (col) #1=1 ("disabled index (col)"), new element #2=w812, index (col) #2=2 ("disabled index (col)"), new element #3=w813, index (col) #3=3 ("disabled index (col)"), new element #4=w816, index (col) #4=4 ("disabled index (col)")) -> (w821:string[][])  [unwired: 4 in]
        n404 = local write "Cycle Pattern"(w821) -> ()
      }
      frame "load cycle name" {
        n405 = property on="Cycle Pattern" class="Tbl (strict)"() -> ("EditPos"=w882:T3)  [unwired: 2 in, 2 out]
        n406 = Unbundle By Name(w882) -> ("Row"=w880:i32, "Column"=w879:i32)
        n407 = local read "Cycle Pattern"() -> (w878:string[][])
        n408 = call "SubCycles list.vi"() -> ("Subcycle name"=w881:string)  [unwired: 10 in, 1 out]
        n409 = Replace Array Subset(array=w878, new element=w881, index (row)=w880, index (col)=w879) -> (w877:string[][])
        n410 = local write "Cycle Pattern"(w877) -> ()
      }
      frame "load test array" {
        n411 = local read "Total Test Duration (hrs)"() -> (w890:T8)
        n412 = local read "Cycle Name"() -> (w886:T5)
        n413 = Equal?(x=w886, y="") -> (x = y?=w885:bool)
        n414 = Not Equal?(x=w890, y="0:00:00") -> (x != y?=w884:bool)
        n415 = Or(x=w884, y=w885) -> (x .or. y?=w883:bool)
        n416 = case shown="True" w883 {
          selector: w883 -> [w891 _]
          tunnel: [FALSE TRUE] -> w888
          frame False {
            n417 = case shown="False" w891 {
              frame False {
                n418 = One Button Dialog(message="Incomplete Data!\nReview the cycle pattern!") -> ()  [unwired: 1 in, 1 out]
              }
              frame True {
              }
            }
          }
          frame True {
            w897 = 0.0 ("default (0 I32)")
            n419 = local read "Cycle Name"() -> (w912:T5)
            n420 = Concatenate Strings("C:\\Setup Files\\Cycles Folder\\", w912, ".eyec" ("string")) -> (w910:string)
            n421 = String To Path(string=w910) -> (path=w911:path)
            n422 = local read "Total Number of Cycles"() -> (w908:T1)
            n423 = call-poly <vilib>:"Read From Spreadsheet File.vi"("file path (dialog if empty)"=w911) -> ("first row"=w894:string[])  [unwired: 6 in, 4 out]
            n424 = call "Remove names.vi"("Array in"=w894) -> ("Array out"=w903:string[])  [unwired: 10 in]
            n425 = Index Array(array=w894, index #1=14 ("index"), index #2=15 ("index")) -> (element #1=w899:string, element #2=w895:string)
            n426 = Number To Decimal String(number="Ageing Gas") -> (decimal integer string=w907:string)  [unwired: 1 in]
            n427 = Number To Decimal String(number=w908) -> (decimal integer string=w906:string)  [unwired: 1 in]
            n428 = Decimal String To Number(string=w895, default (0L)=w897) -> (number=w896:dbl)  [unwired: 1 in, 1 out]
            n429 = Decimal String To Number(string=w899, default (0L)=w897) -> (number=w898:dbl)  [unwired: 1 in, 1 out]
            n430 = property on="Inlet temp Age" class="DigNum (strict)"("Value"=w898) -> ()  [unwired: 2 in, 2 out]
            n431 = property on="Flow rate Age" class="DigNum (strict)"("Value"=w896) -> ()  [unwired: 2 in, 2 out]
            n432 = Build Array (concatenate)(w907, w906, w903) -> (w902:string[])
            n433 = shared-variable "NI-cRIO9074-018C1D8D\\Library 1.lvlib\\Ageing Variables"(w902) -> ()  [unwired: 1 in, 1 out]
          }
        }
        "Test Compiled" <- w888
      }
      frame "convert to num" {
        n434 = local read "EditPos Subc"() -> (w917:T3)
        n435 = Unbundle By Name(w917) -> ("Row"=w918:i32, "Column"=w915:i32)
        n436 = Equal?(x=w915, y=7) -> (x = y?=w914:bool)
        n437 = case shown="False" w914 {
          tunnel: w918 -> [_ w923]
          tunnel: w915 -> [_ w921]
          tunnel: w917 -> [_ _]
          frame True {
          }
          frame False {
            n438 = local read "Sub-Cycle Pattern"() -> (w920:string[][])
            n439 = call "Conv to num.vi"("Column"=w921, "Row"=w923, "Array"=w920) -> ("result string"=w922:string)  [unwired: 8 in]
            n440 = Replace Array Subset(array=w920, new element=w922, index (row)=w923, index (col)=w921) -> (w919:string[][])
            n441 = local write "Sub-Cycle Pattern"(w919) -> ()
          }
        }
      }
      frame "check scycle name" {
        n442 = local read "Sub-Cycle Name"() -> (w924:T5)
        n443 = call <vilib>:"Search and Replace Pattern.vi"("string"=w924, "regular expression (\"\")"="[^0-9a-zA-Z ]" ("format string"), "replace string (\"\")"="", "replace all? (F)"=TRUE) -> ("result string"=w930:string)  [unwired: 1 in, 1 out]
        n444 = Not Equal?(x=w930, y=w924) -> (x != y?=w929:bool)
        n445 = case shown="False" w929 {
          tunnel: w930 -> [w931 w932]
          tunnel: [w931 w932] -> w925
          frame False {
          }
          frame True {
            n446 = One Button Dialog(message="Unsuitable character for the file name!") -> ()  [unwired: 1 in, 1 out]
          }
        }
        n447 = local write "Sub-Cycle Name"(w925) -> ()
      }
      frame "check cycle name" {
        n448 = local read "Cycle Name"() -> (w934:T5)
        n449 = call <vilib>:"Search and Replace Pattern.vi"("string"=w934, "regular expression (\"\")"="[^0-9a-zA-Z ]" ("format string"), "replace string (\"\")"="", "replace all? (F)"=TRUE) -> ("result string"=w940:string)  [unwired: 1 in, 1 out]
        n450 = Not Equal?(x=w940, y=w934) -> (x != y?=w939:bool)
        n451 = case shown="False" w939 {
          tunnel: w940 -> [w941 w942]
          tunnel: [w941 w942] -> w935
          frame False {
          }
          frame True {
            n452 = One Button Dialog(message="Unsuitable character for the file name!") -> ()  [unwired: 1 in, 1 out]
          }
        }
        n453 = local write "Cycle Name"(w935) -> ()
      }
      frame "Multigas connect" {
        n454 = flat-sequence {
          frame #0 {
            "Connected?" <- TRUE
          }
        }
      }
      frame "Multigas disconnect" {
      }
    }
    n455 = local read "stop 2"() -> (w330:bool)
  }
  n456 = disable-structure shown="Disabled" {
    frame Disabled {
      n457 = while {
        tunnel: [w983] -> w968
        tunnel: [w982] -> w967
        stop <- w979 stop-if-true
        n458 = TCP Open Connection(address="192.168.1.3", remote port or service name=u16 7700) -> (connection ID=w983:refnum<k5>, error out=w982:errorcluster)  [unwired: 3 in]
        n459 = Unbundle By Name(w982) -> ("status"=w984:bool)
        n460 = Not(x=w984) -> (.not. x?=w980:bool)
        n461 = Or(x=w980, y="stop TCP") -> (x .or. y?=w979:bool)
      }
      n462 = Concatenate Strings("\r", "\n") -> (w956:string)
      n463 = Concatenate Strings("MSSM,0,1,1" ("data in"), w956) -> (w963:string)
      n464 = TCP Write(connection ID=w968, data in=w963, error in (no error)=w967) -> (connection ID out=w971:refnum<k5>, error out=w972:errorcluster)  [unwired: 1 in, 1 out]
      n465 = Concatenate Strings("MSMD,1,7,1,1,1,1,2,1,1,3,1,1,4,1,1,5,1,1,6,1,1,7,1" ("data in"), w956) -> (w958:string)
      n466 = TCP Write(connection ID=w971, data in=w958, error in (no error)=w972) -> (connection ID out=w969:refnum<k5>, error out=w970:errorcluster)  [unwired: 1 in, 1 out]
      n467 = Concatenate Strings("MSTT,1,0" ("string"), w956) -> (w957:string)
      n468 = TCP Write(connection ID=w969, data in=w957, error in (no error)=w970) -> (connection ID out=w955:refnum<k5>, error out=w954:errorcluster)  [unwired: 1 in, 1 out]
      n469 = UDP Open(9:500 ("timeout ms (25000)"), 11:u16 7701 ("port")) -> ()  [unwired: 3 in, 3 out]
      n470 = UDP Read(timeout ms (25000)=500) -> (data out=w946:string)  [unwired: 3 in, 4 out]
      n471 = while {
        shift-right: [w975] -> _
        shift-left: w946 -> [w978]
        tunnel: [w976] -> w947 mode=indexing
        stop <- w973 stop-if-true
        n472 = Search/Split String(string=w978, search string/char (-)=",") -> (substring before match=w976:string, match + rest of string=w975:string)  [unwired: 1 in, 1 out]
        n473 = String Length(string=w975) -> (length=w974:i32)
        n474 = Equal To 0?(x=w974) -> (x = 0?=w973:bool)
      }
      n475 = call "7170string to array.vi"("Array in"=w947) -> ()  [unwired: 4 in, 1 out]
      n476 = UDP Close() -> ()  [unwired: 2 in, 2 out]
      n477 = Concatenate Strings("MSTP,0,0" ("string"), "\r", "\n") -> (w950:string)
      n478 = TCP Write(data in=w950) -> (connection ID out=w952:refnum<k5>, error out=w953:errorcluster)  [unwired: 3 in, 1 out]
      n479 = TCP Close Connection(connection ID=w952, error in (no error)=w953) -> ()  [unwired: 1 in, 2 out]
    }
    frame Enabled {
    }
  }
  n480 = while {
    tunnel: w35 -> [w991]
    shift-right: [w989] -> _
    shift-left: _ -> [w988]
    stop <- w987 stop-if-true
    n481 = event shown="[12] \"Cycle Pattern\": Mouse Up;  \"Cycle Pattern\": Value Change" {
      selector: _ -> [_ _ _ _ _ _ _ _ _ _ _ _ _ _ _ _ _ _ _ _ _ _ _ _ _ _ _ _]
      dyn-events: _ -> [_ _ _ _ _ _ _ _ _ _ _ _ _ _ _ _ _ _ _ _ _ _ _ _ _ _ _ _]
      timeout: 100 -> [_ _ _ _ _ _ _ _ _ _ _ _ _ _ _ _ _ _ _ _ _ _ _ _ _ _ _ _]
      tunnel: w991 -> [w994 w996 _ w1005 w1013 w1020 w1027 w1038 w1042 w1053 w1058 w1061 w1066 w1088 w1096 w1097 _ _ _ _ w1141 w1151 w1173 w1191 _ w1205 _ _]
      tunnel: [w992 w995 _ w1006 w1012 w1019 w1026 w1037 w1040 w1048 w1055 w1060 w1064 w1085 _ _ _ _ _ _ _ _ _ _ _ _ _ _] -> w989
      tunnel: w988 -> [w992 w995 _ w1006 w1012 w1019 w1025 w1037 w1040 w1048 w1055 w1060 w1064 w1085 _ _ _ _ _ _ _ _ _ _ _ _ _ _]
      tunnel: [_ _ w998 _ _ _ _ _ _ _ _ _ _ _ _ _ _ _ _ _ _ _ _ _ _ _ _ _] -> w987
      event Timeout {
        n482 = event-data() -> ()  [unwired: 1 in, 2 out]
        n483 = Enqueue Element(queue=w994, element=Control_3."main" ("Enum")) -> ()  [unwired: 2 in, 3 out]
      }
      event "Clear subcycle": Value Change {
        n484 = event-data() -> ()  [unwired: 1 in, 5 out]
        n485 = Enqueue Element(queue=w996, element=Control_3."clear table 1" ("Enum")) -> ()  [unwired: 2 in, 3 out]
      }
      event Panel Close? {
        n486 = event-data() -> ()  [unwired: 1 in, 3 out]
        n487 = Two Button Dialog(message="This command will close Eyecat!\nDo you wish to continue?", 1:"No" ("F button name (\"Cancel\")"), 2:"Yes" ("T button name (\"OK\")")) -> (T button?=w998:bool)
        n488 = Not(x=w998) -> (.not. x?=w999:bool)
        n489 = event-data("Discard?"=w999) -> ()  [unwired: 1 in, 1 out]
      }
      event "Save sCycle": Value Change {
        n490 = event-data() -> ()  [unwired: 1 in, 5 out]
        n491 = local read "Sub-Cycle Pattern"() -> (w1003:string[][])
        n492 = call "Time column check.vi"("Array"=w1003) -> ("Mistake?"=w1004:bool)  [unwired: 10 in]
        n493 = case shown="False" w1004 {
          tunnel: w1005 -> [w1007 _]
          frame False {
            n494 = Enqueue Element(queue=w1007, element=Control_3."save subc") -> (queue out=w1009:refnum<queue>)  [unwired: 2 in, 2 out]
            n495 = Enqueue Element(queue=w1009, element=Control_3."update list 1") -> ()  [unwired: 2 in, 3 out]
          }
          frame True {
            n496 = One Button Dialog(message="The time sequence is incorrect!\nReview and save again!") -> ()  [unwired: 1 in, 1 out]
          }
        }
      }
      event "Load sCycle": Value Change {
        n497 = event-data() -> ()  [unwired: 1 in, 5 out]
        n498 = Enqueue Element(queue=w1013, element=Control_3."load subc") -> ()  [unwired: 2 in, 3 out]
      }
      event "Delete sCycle": Value Change {
        n499 = event-data() -> ()  [unwired: 1 in, 5 out]
        n500 = Enqueue Element(queue=w1020, element=Control_3."delete subc") -> (queue out=w1022:refnum<queue>)  [unwired: 2 in, 2 out]
        n501 = Enqueue Element(queue=w1022, element=Control_3."update list 1") -> (queue out=w1018:refnum<queue>)  [unwired: 2 in, 2 out]
        n502 = Enqueue Element(queue=w1018, element=Control_3."update Cycle pattern ") -> (queue out=w1015:refnum<queue>)  [unwired: 2 in, 2 out]
        n503 = Enqueue Element(queue=w1015, element=Control_3."Total time calc") -> ()  [unwired: 2 in, 3 out]
      }
      event "Sub-Cycle Pattern": Mouse Down; "Sub-Cycle Pattern": Value Change {
        n504 = event-data() -> ()  [unwired: 1 in, 3 out]
        n505 = property on="Sub-Cycle Pattern" class="Tbl (strict)"() -> ("EditPos"=w1026:T3)  [unwired: 2 in, 2 out]
        n506 = Unbundle By Name(w1026) -> ("Row"=w1028:i32)  [unwired: 1 out]
        n507 = Less?(x=w1028, y=30) -> (x < y?=w1030:bool)
        n508 = case shown="True" w1030 {
          tunnel: w1027 -> [_ w1035]
          frame False {
            n509 = One Button Dialog(message="This table is limited to 30 entries!") -> ()  [unwired: 1 in, 1 out]
          }
          frame True {
            n510 = Enqueue Element(queue=w1035, element=Control_3."convert to num") -> (queue out=w1034:refnum<queue>)  [unwired: 2 in, 2 out]
            n511 = Enqueue Element(queue=w1034, element=Control_3."calc HC CO") -> ()  [unwired: 2 in, 3 out]
          }
        }
        "EditPos Subc" <- w1025
        "Flag1" <- TRUE
      }
      event "Clear Cycle Pattern": Value Change {
        n512 = event-data() -> ()  [unwired: 1 in, 5 out]
        n513 = Enqueue Element(queue=w1038, element=Control_3."clear table 2" ("Enum")) -> ()  [unwired: 2 in, 3 out]
        n514 = local write "Test Compiled"(FALSE ("Test Compiled")) -> ()
      }
      event "Save Cycle": Value Change {
        n515 = event-data() -> ()  [unwired: 1 in, 5 out]
        n516 = Enqueue Element(queue=w1042, element=Control_3."update Cycle pattern ") -> (queue out=w1041:refnum<queue>)  [unwired: 2 in, 2 out]
        n517 = Enqueue Element(queue=w1041, element=Control_3."save cycle") -> (queue out=w1045:refnum<queue>)  [unwired: 2 in, 2 out]
        n518 = Enqueue Element(queue=w1045, element=Control_3."update list 2") -> ()  [unwired: 2 in, 3 out]
      }
      event "Load Cycle": Value Change {
        n519 = event-data() -> ()  [unwired: 1 in, 5 out]
        n520 = Enqueue Element(queue=w1053, element=Control_3."load cycle") -> (queue out=w1051:refnum<queue>)  [unwired: 2 in, 2 out]
        n521 = Enqueue Element(queue=w1051, element=Control_3."update Cycle pattern ") -> (queue out=w1050:refnum<queue>)  [unwired: 2 in, 2 out]
        n522 = local write "Test Compiled"(FALSE ("Test Compiled")) -> ()
        n523 = Enqueue Element(queue=w1050, element=Control_3."Total time calc") -> ()  [unwired: 2 in, 3 out]
      }
      event "Delete Cycle": Value Change {
        n524 = event-data() -> ()  [unwired: 1 in, 5 out]
        n525 = Enqueue Element(queue=w1058, element=Control_3."delete cycle") -> (queue out=w1057:refnum<queue>)  [unwired: 2 in, 2 out]
        n526 = Enqueue Element(queue=w1057, element=Control_3."update list 2") -> ()  [unwired: 2 in, 3 out]
      }
      event Value Change {
        n527 = event-data() -> ()  [unwired: 1 in, 5 out]
        n528 = Enqueue Element(queue=w1061, element=Control_3."Total time calc") -> ()  [unwired: 2 in, 3 out]
      }
      event "Cycle Pattern": Mouse Up; "Cycle Pattern": Value Change {
        n529 = event-data() -> ()  [unwired: 1 in, 3 out]
        n530 = property on="Cycle Pattern" class="Tbl (strict)"() -> ("EditPos"=w1068:T3)  [unwired: 2 in, 2 out]
        n531 = Unbundle By Name(w1068) -> ("Row"=w1065:i32, "Column"=w1070:i32)
        n532 = Less?(x=w1065, y=30) -> (x < y?=w1069:bool)
        n533 = case shown="True" w1069 {
          tunnel: w1070 -> [_ w1072]
          tunnel: w1066 -> [_ w1075]
          frame False {
            n534 = One Button Dialog(message="This table is limited to 30 entries!") -> ()  [unwired: 1 in, 1 out]
          }
          frame True {
            n535 = Equal?(x=w1072, y=1) -> (x = y?=w1076:bool)
            n536 = case shown="True" w1076 {
              tunnel: w1075 -> [w1079 w1082]
              tunnel: [w1078 w1081] -> w1074
              frame False {
                n537 = Enqueue Element(queue=w1079, element=Control_3."update Cycle pattern ") -> (queue out=w1078:refnum<queue>)  [unwired: 2 in, 2 out]
              }
              frame True {
                n538 = Enqueue Element(queue=w1082, element=Control_3."load cycle name") -> (queue out=w1081:refnum<queue>)  [unwired: 2 in, 2 out]
              }
            }
            n539 = Enqueue Element(queue=w1074, element=Control_3."Total time calc") -> ()  [unwired: 2 in, 3 out]
          }
        }
        "Flag 2" <- TRUE
      }
      event "Compile Test Button": Value Change {
        n540 = event-data() -> ()  [unwired: 1 in, 5 out]
        n541 = local read "Flag 2"() -> (w1084:bool)
        n542 = case shown="True" w1084 {
          tunnel: w1088 -> [w1089 w1093]
          tunnel: [w1089 w1090] -> w1086
          frame False {
          }
          frame True {
            n543 = Enqueue Element(queue=w1093, element=Control_3."save cycle") -> (queue out=w1091:refnum<queue>)  [unwired: 2 in, 2 out]
            n544 = Enqueue Element(queue=w1091, element=Control_3."update list 2") -> (queue out=w1090:refnum<queue>)  [unwired: 2 in, 2 out]
          }
        }
        n545 = Enqueue Element(queue=w1086, element=Control_3."load test array") -> ()  [unwired: 2 in, 3 out]
      }
      event Value Change {
        n546 = event-data() -> ()  [unwired: 1 in, 5 out]
        n547 = Enqueue Element(queue=w1096, element=Control_3."check scycle name") -> ()  [unwired: 2 in, 3 out]
      }
      event Value Change {
        n548 = event-data() -> ()  [unwired: 1 in, 5 out]
        n549 = Enqueue Element(queue=w1097, element=Control_3."check cycle name") -> ()  [unwired: 2 in, 3 out]
      }
      event Value Change {
        n550 = event-data() -> ()  [unwired: 1 in, 5 out]
        n551 = Square(x="Sample Diameter (mm)") -> (x^2=w1106:T1)
        n552 = Compound Arithmetic op=MULTIPLY(w1106, "Sample Length (mm)", "Number of Samples", 3.141592653589793) -> (w1105:T1)
        n553 = Divide(x=w1105, y=4000000.0) -> (x/y=→"Sample Volume (litres)":T1)
      }
      event Value Change {
        # "O2Eq"
        n554 = event-data() -> ()  [unwired: 1 in, 5 out]
        n555 = local write "Inlet LAMBDA"("Inlet LAMBDA") -> ()
        n556 = local write "Inlet O2 (%)"("Inlet O2 (%)") -> ()
        n557 = Decrement(x="Inlet LAMBDA") -> (x-1=w1121:T1)
        n558 = Multiply(x=4.76, y="Inlet LAMBDA") -> (x*y=w1117:T1)
        n559 = Multiply(x=w1121, y=100.0) -> (x*y=w1119:T1)
        n560 = Add(x=0.33, y=w1117) -> (x+y=w1115:T1)
        n561 = Divide(x=w1119, y=w1115) -> (x/y=w1114:T1)
        n562 = Subtract(x="Inlet O2 (%)", y=w1114) -> (x-y=w1112:T1)
        n563 = Multiply(x=w1112, y=2.0) -> (x*y=→"CO Theory (%)":T1)
        n564 = Divide(x=w1112, y=4.5) -> (x/y=→"HC Theory (%)":T1)
      }
      event Value Change {
        n565 = event-data() -> ()  [unwired: 1 in, 5 out]
        n566 = local write "NO ppm Loff"("NO ppm Loff") -> ()
        n567 = local write "NO:CO Ratio"("NO:CO Ratio") -> ()
        n568 = Divide(x="NO ppm Loff", y=T1 10000.0) -> (x/y=w1124:T1)
        n569 = Multiply(x="NO:CO Ratio", y=w1124) -> (x*y=→"CO Theory (%)":T1)
      }
      event Value Change {
        n570 = event-data() -> ()  [unwired: 1 in, 5 out]
        n571 = local read "Sample Volume (litres)"() -> (w1129:T7)
        n572 = Equal?(x=w1129, y=0.0) -> (x = y?=w1128:bool)
        n573 = case shown="False" w1128 {
          tunnel: w1129 -> [w1134 _]
          tunnel: "Test Flow Rate(g/s)" -> [w1131 _]
          frame False {
            w1136 = 60.0 ("y")
            n574 = Multiply(x=w1131, y=w1136) -> (x*y=w1138:T1)
            n575 = Divide(x=w1138, y=1.2) -> (x/y=w1133:T1)
            "Vol Flow @ STP (l/min)" <- w1133
            n576 = Multiply(x=w1133, y=w1136) -> (x*y=w1135:T1)
            n577 = Divide(x=w1135, y=w1134) -> (x/y=→"Space Velocity (h-1)":T1)
          }
          frame True {
            n578 = One Button Dialog(message="Review sample specification first!") -> ()  [unwired: 1 in, 1 out]
          }
        }
      }
      event "Execute Leak Test Button": Value Change {
        n579 = event-data() -> ()  [unwired: 1 in, 5 out]
        n580 = flat-sequence {
          tunnel: w1141 -> [w1144]
          tunnel: [w1144] -> w1140
          tunnel: w1140 -> [w1147]
          frame #0 {
            n581 = local write "Test number"(u16 5) -> ()
            n582 = local write "Enum 1"(u16 3 ("Test number")) -> ()
          }
          frame #1 {
            n583 = Enqueue Element(queue=w1147, element=Control_3."main" ("Enum")) -> (queue out=w1145:refnum<queue>)  [unwired: 2 in, 2 out]
            n584 = Enqueue Element(queue=w1145, element=Control_3."start test" ("Enum")) -> ()  [unwired: 2 in, 3 out]
          }
        }
      }
      event "Start Test Button": Value Change {
        n585 = event-data() -> ()  [unwired: 1 in, 5 out]
        n586 = flat-sequence {
          tunnel: w1151 -> [w1154]
          tunnel: [w1154] -> w1150
          tunnel: w1150 -> [w1158]
          tunnel: [w1155] -> w1149
          tunnel: w1149 -> [w1166]
          frame #0 {
            n587 = local write "Enum 1"(u16 1 ("Test number")) -> ()
            "Test number" <- "Select Test Type"
          }
          frame #1 {
            n588 = Two Button Dialog(message="Do you wish to connect to\nthe external analyser?   \n") -> (T button?=w1156:bool)  [unwired: 2 in]
            n589 = case shown="True" w1156 {
              tunnel: w1158 -> [w1159 w1161]
              tunnel: [w1159 w1160] -> w1155
              frame False {
              }
              frame True {
                n590 = Enqueue Element(queue=w1161, element=Control_3."Multigas connect" ("Enum")) -> (queue out=w1160:refnum<queue>)  [unwired: 2 in, 2 out]
              }
            }
          }
          frame #2 {
            n591 = Enqueue Element(queue=w1166, element=Control_3."main" ("Enum")) -> (queue out=w1164:refnum<queue>)  [unwired: 2 in, 2 out]
            n592 = property on="Stop Test Button" class="Bool"("DisabledEnum"=T13."Enabled" ("Disabled")) -> ()  [unwired: 2 in, 2 out]
            n593 = Enqueue Element(queue=w1164, element=Control_3."start test" ("Enum")) -> ()  [unwired: 2 in, 3 out]
          }
        }
      }
      event "Stop Test Button": Value Change {
        n594 = event-data() -> ()  [unwired: 1 in, 5 out]
        n595 = flat-sequence {
          tunnel: w1173 -> [w1175]
          tunnel: [w1175] -> w1172
          tunnel: [w1174] -> w1170
          tunnel: w1172 -> [w1179]
          tunnel: [w1178] -> w1171
          tunnel: w1170 -> [w1178]
          tunnel: [w1177] -> w1169
          tunnel: w1171 -> [w1183]
          tunnel: w1169 -> [w1182]
          tunnel: [T13."Disabled and Grayed Out" ("Disabled")] -> w1168
          frame #0 {
            n596 = local read "Connected?"() -> (w1174:bool)
            n597 = local write "Stop Cmd"(T1 1.0 ("Stop Cmd")) -> ()
          }
          frame #1 {
            n598 = Enqueue Element(queue=w1179, element=Control_3."main" ("Enum")) -> (queue out=w1177:refnum<queue>)  [unwired: 2 in, 2 out]
          }
          frame #2 {
            n599 = case shown="True" w1183 {
              tunnel: w1182 -> [w1184 w1187]
              tunnel: [w1184 w1186] -> _
              frame False {
              }
              frame True {
                n600 = local write "Connected?"(FALSE ("Connected?")) -> ()
                n601 = Enqueue Element(queue=w1187, element=Control_3."Multigas disconnect" ("Enum")) -> (queue out=w1186:refnum<queue>)  [unwired: 2 in, 2 out]
              }
            }
          }
        }
        n602 = property on="Stop Test Button" class="Bool"("DisabledEnum"=w1168) -> ()  [unwired: 2 in, 2 out]
      }
      event "Stopped?": Value Change {
        n603 = event-data() -> ()  [unwired: 1 in, 5 out]
        n604 = flat-sequence {
          tunnel: w1191 -> [w1195]
          tunnel: [w1194] -> w1190
          tunnel: [w1193] -> w1189
          tunnel: w1190 -> [w1197]
          tunnel: w1189 -> [w1196]
          frame #0 {
            n605 = local read "Connected?"() -> (w1193:bool)
            n606 = Enqueue Element(queue=w1195, element=Control_3."main" ("Enum")) -> (queue out=w1194:refnum<queue>)  [unwired: 2 in, 2 out]
          }
          frame #1 {
            n607 = case shown="True" w1196 {
              tunnel: w1197 -> [_ w1198]
              frame False {
              }
              frame True {
                n608 = local write "Connected?"(FALSE ("Connected?")) -> ()
                n609 = Enqueue Element(queue=w1198, element=Control_3."Multigas disconnect" ("Enum")) -> ()  [unwired: 2 in, 3 out]
              }
            }
          }
        }
      }
      event "Alarm ack": Value Change {
        # "system alarm - set to off"
        n610 = event-data() -> ()  [unwired: 1 in, 5 out]
        n611 = local write "Acknowledge"(TRUE ("Acknowledge")) -> ()
        n612 = property on="Soft Alarm" class="Bool (strict)"("Value"=FALSE ("Acknowledge")) -> ()  [unwired: 2 in, 2 out]
        n613 = property on="Alarm ack" class="Bool"("DisabledEnum"=T13."Disabled and Grayed Out" ("Disabled")) -> ()  [unwired: 2 in, 2 out]
      }
      event "Purge System": Value Change {
        n614 = event-data() -> ()  [unwired: 1 in, 5 out]
        n615 = flat-sequence {
          tunnel: w1205 -> [w1207]
          tunnel: [w1207] -> w1204
          tunnel: w1204 -> [w1208]
          frame #0 {
            n616 = local write "Enum 1"(u16 4 ("Test number")) -> ()
          }
          frame #1 {
            n617 = Enqueue Element(queue=w1208, element=Control_3."start test" ("Enum")) -> ()  [unwired: 2 in, 3 out]
          }
        }
      }
      event "Clear log": Value Change {
        n618 = event-data() -> ()  [unwired: 1 in, 5 out]
        n619 = local write "Table"(string[][] [] ("Table")) -> ()
      }
      event "Advanced settings": Value Change {
        # "To be updated"
        # "SO2 conc\nNOx conc\nCO conc\nHC conc\nBleed ratio N2\nBleed ratio CO2"
        n620 = event-data() -> ()  [unwired: 1 in, 5 out]
        n621 = call "Advanced settings MAX.vi"() -> ("output cluster"=→"output cluster":T14)  [unwired: 1 in]
      }
    }
    "stop 2" <- w987
  }
  n622 = local write "stop 2"(w9) -> ()
  n623 = node-c288(w6) -> ()  [unwired: 1 out]
  "Table" <- string[][] [] ("Table")
